vi "Plotter_General.vi"() -> ()   [LabVIEW 2013]
uses:
  Shared/MySQL/Preset Query Enum.ctl
  plotter setup cluster.ctl
  <vilib>/Analysis/NI_AALBase.lvlib
  <vilib>/Analysis/1siggen.llb/Ramp Pattern by Samples.vi
  <vilib>/Utility/tcp.llb/UDP Multicast Read-Only Open.vi
  General-Controler/panel position.ctl
panel:
  in  "STOP button":bool
  in  "shot# 3":i32
  out "error out 3":errorcluster
  out "TCP Ports":refnum<k5>[](array[refnum])
  in  "Device name":string
  in  "shot #":i32
  in  "data string":string
  in  "data string 2":string
  in  "shot # 2":i32
  in  "Device name 2":string
  out "subscribe command":string
  out "size(s)":i32
  out "appended array":string[](array[string])
  out "y2":dbl[](array[numeric])
  out "y1":dbl[](array[numeric])
  out "error out 4":errorcluster
  out "x":dbl[](array[numeric])
  out "portrsvvv":string[](array[string])
  out "ipjjj":string[](array[string])
  out "IPs":string[](array[string])
  out "udp ports to listen to":string[](array[string])
  in  "TCP Open timeout ms":i32=1000
  out "TCP scan error out":errorcluster
  out "ScanData to receive":string[][](array[string])
  out "error out":errorcluster
  in  "Cluster":T1
  out "appargs":string[](array[string])
  out "plotter details":string[][](array[string])
  out "expt":string
  out "Mcast Data":string
  out "TDMS file path":path
  in  "Tab Control 2":T2(tab)
  out "parameters to get":string[][](array[string])
  out "devices to get data from":string[](array[string])
  out "Axis Name List":string[](array[string])
  out "All Devices Core Info":string[][](array[string])
  out "UDP Mcast Error":errorcluster
  in  "Tab Control":T3(tab)=enum."Binned Plot"
  out "xy graph":cluster{dbl[], dbl[]}[](graph)
  out "LHS sigma":dbl format="%_4p"
  out "LHS mean":dbl format="%_4p"
  out "RHS mean":dbl format="%_4p"
  out "RHS sigma":dbl format="%_4p"
  out "Screen\nPosition":cluster{"Left":i16, "Top":i16}
  out "plotter#":string
  out "Scan number":string
  out "xy graph bin":cluster{dbl[], dbl[]}[](graph)=[{[5.5, 15.5, 25.5, 35.5, 45.5, 55.5, 0.0], [0.1, 0.1, 0.15, 0.15, 0.2, 0.2, 0.0]}, {[5.5, 5.5, nan, 15.5, 15.5, nan, 25.5, 25.5, nan, 35.5, 35.5, nan, 45.5, 45.5, nan, 55.5, 55.5, nan, 0.0, 0.0, nan], [0.1, 0.1, nan, 0.1, 0.1, nan, 0.15, 0.15, nan, 0.15, 0.15, nan, 0.2, 0.2, nan, 0.2, 0.2, nan, 0.0, 0.0, nan]}, {[5.5, 15.5, 25.5, 35.5, 45.5, 55.5, 0.0], [5.5, 15.5, 25.5, 35.5, 45.5, 55.5, 0.0]}, {[5.5, 5.5, nan, 15.5, 15.5, nan, 25.5, 25.5, nan, 35.5, 35.5, nan, 45.5, 45.5, nan, 55.5, 55.5, nan, 0.0, 0.0, nan], [3.0, 8.0, nan, 13.0, 18.0, nan, 23.0, 28.0, nan, 33.0, 38.0, nan, 43.0, 48.0, nan, 53.0, 58.0, nan, 0.0, 0.0, nan]}]
  in  "replot":bool
  out "Experiment":u16(ring) items=["Bella", "DataLogging", "HeaterTest", "Lanex Bella", "Plasma2", "Test"]
  out "Current State":string
  out "Mcast Path Data":string
  in  "FilePath":bool
  in  "file path":path
  in  "X Axis":u16(ring)=1 items=["DateTime DateTime shot #", "DateTime Timestamp", "Rep Rate Rep Rate shot #", "Rep Rate Hz"]
  in  "Y Axis":u16(ring) items=["DateTime DateTime shot #", "DateTime Timestamp", "Rep Rate Rep Rate shot #", "Rep Rate Hz"]
  in  "Y Axis 2":u16(ring) items=["DateTime DateTime shot #", "DateTime Timestamp", "Rep Rate Rep Rate shot #", "Rep Rate Hz"]
  out "device data Spreadsheet format":string[][](array[string])
  in  "Left":i16=25
  in  "Top":i16=75
  in  "expt_Plotteridfor vi mode":string="38"
  in  "timeout ms":i32=1000
  out "Actual expt_plotter.id":string
  out "x axis name":string
  out "ScanStart ExptName":string
  out "Y Axis Default name":string
  out "MC_IP":string
  out "Path used":path
  out "error out 2":errorcluster
  out "ScanStatus":string
  in  "data out 1":string
  in  "data out 3":string
  in  "data out 2":string
  out "shotoverride":bool
  in  "shot#":i32
  in  "shot# 2":i32
  out "error out 5":errorcluster
  # "Plotter"
  # "17 Fake cam 1 to 5"
  # "15"
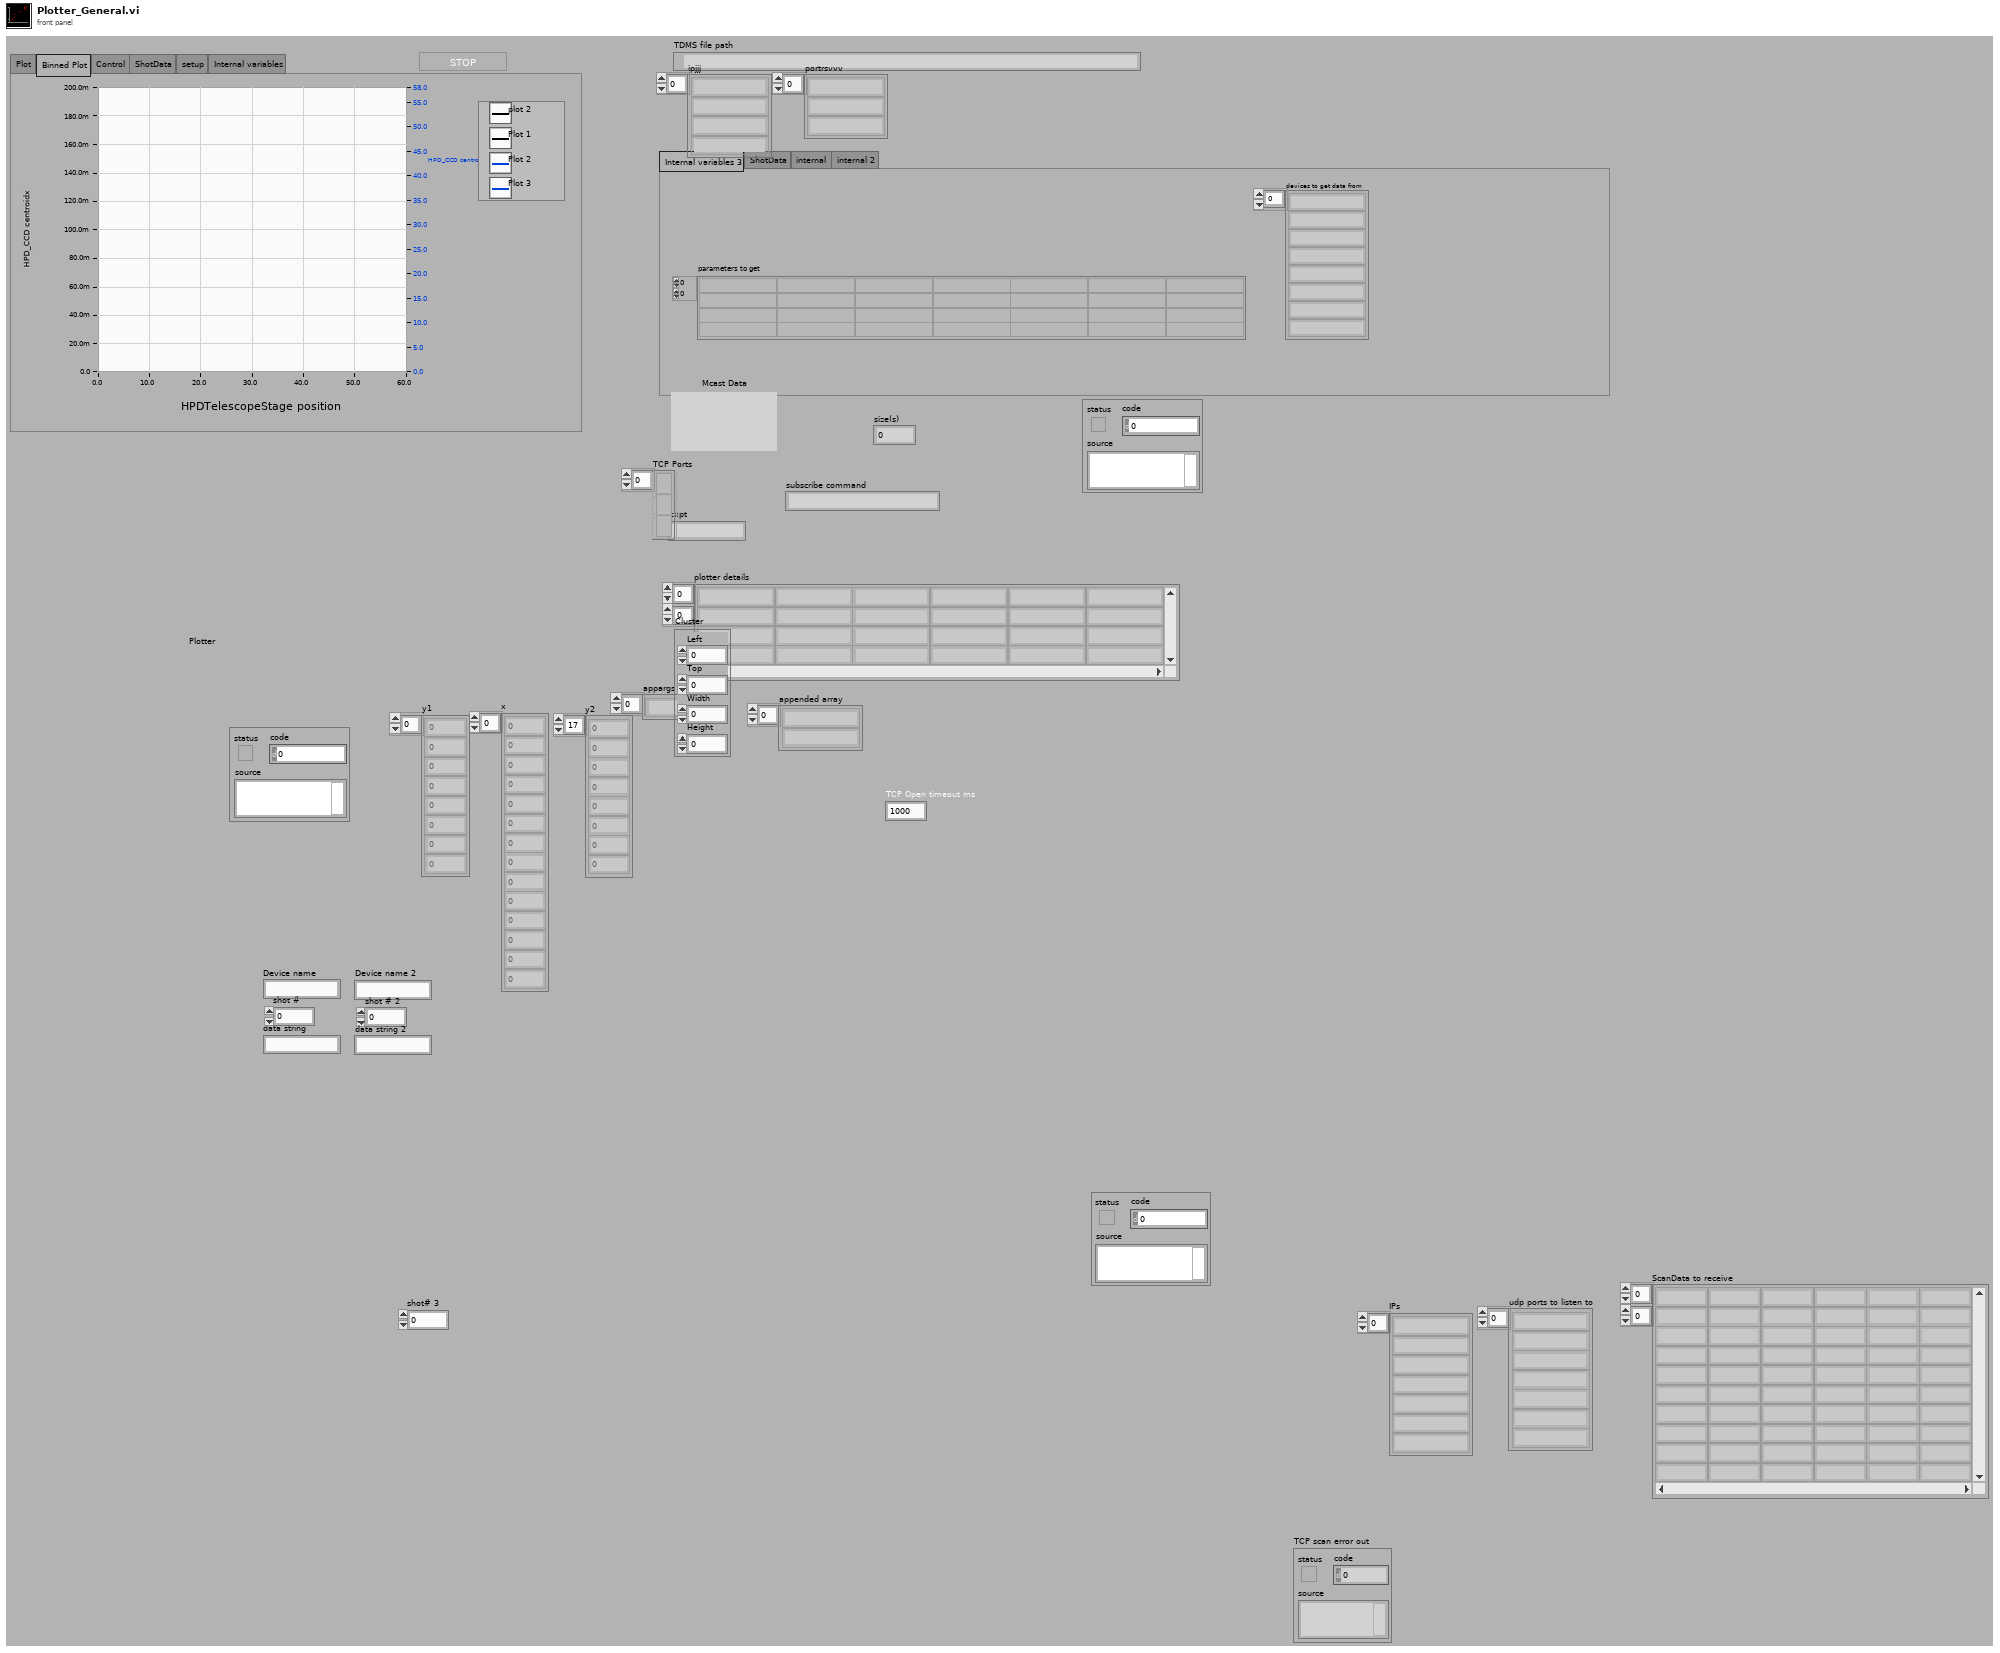
[diagram p1: front panel]
types:
  T1 = typedef "panel position.ctl" = cluster{"Left":i16, "Top":i16, "Width":u32, "Height":u32}
  T2 = enum32{"Internal variables 3", "ShotData", "internal", "internal 2"}
  T3 = enum32{"Plot", "Binned Plot", "Control", "ShotData", "setup", "Internal variables"}
  T4 = typedef "Plotter FGV cluster control.ctl" = cluster{"Multicast Address":string, "Plotter Busy":bool, "Plotter Exit":bool, "Mcast Port":u16}
  T5 = enum32{"invalid app kind", "Development System", "Run Time System", "Student Edition", "Embedded LabVIEW", "Evaluation", "Custom"}
  T6 = enum32{"Invalid", "Standard", "Closed", "Hidden", "Minimized", "Maximized"}
  T7 = typedef "Preset Query Enum.ctl" = enum16{"Get Locations", "Get all IPs and MACs", "Get classes", "Get expt variables to set at scanstart for particular device", "Get expt devices and variables with start values", "Get expt devices and variables (with data to get)", "Get expt devices with data to get", "Get Expt devices and GUIs", "Get all devices basic properties", "Get Virtual Devices Core Info", "Get Expt names", "Get experiment basic properties", "Get experiment alarm variables", "Get MC Ports", "Get device network comm port", "Get devicetype lvclass path", "Get basic device properties", "Get Init Order", "Get all setable variables of a device", "Get device variable aliases", "Get force values of all settable variables", "Get all variables of a devicetype", "Get all variables of a device", "Get plotter details", "Get Saved Scans", "Get Scan Info", "GetGeneralGUIs", "Get expt for plotter", "Get plotter IDs from expt", "Get all devices", "Get all Virtual Devices", "Get all aliases", "Get variable and device info for Virtual Device", "GetItemLocatorIP", "Get IPs for GUIs", "Get DeviceType from Device", "GetLocalPortRange", "GetDevicePresetVariables", "Get Device Configuration", "GetAllPresetNames", "GetAllConfigurationNames", "GetPresetDeviceNames"}
  T8 = typedef "plotter setup cluster.ctl" = cluster{"screenx":i16, "screeny":i16, "variable1":string, "variable2":string, "name":string}
  T9 = cluster{"Ring Refnum x":refnum<vi>, "Ring Refnum y":refnum<vi>, "Ring Refnum y 2":refnum<vi>, "XY Graph Refnum":refnum<vi>}
  T10 = cluster{"Core":cluster{"Current VI Reference":refnum<vi>, "Close Panel on Exit?":bool}, "All Devices Core Info":string[][], "Expt Config Files":string[], "Experiment name":string, "ScanData to receive":string[][], "Device Names for scan data":string[], "expt config file array":string[][], "Data titles from config array":string[], "TDMS file path":path, "Plotter setup cluster":T8, "plotter#":string, "bin complete":bool}
  T11 = typedef "LVRectTypeDef.ctl" = cluster{"Left":i16, "Top":i16, "Right":i16, "Bottom":i16}
  T12 = cluster{"TCP Ports":refnum<vi>, "y1":refnum<vi>, "shot#":refnum<vi>, "data out 1":refnum<vi>}
  T13 = cluster{"TCP Ports":refnum<vi>, "y2":refnum<vi>, "shot# 2":refnum<vi>, "data out 2":refnum<vi>}
  T14 = cluster{"TCP Ports":refnum<vi>, "x":refnum<vi>, "shot# 3":refnum<vi>, "data out 3":refnum<vi>}
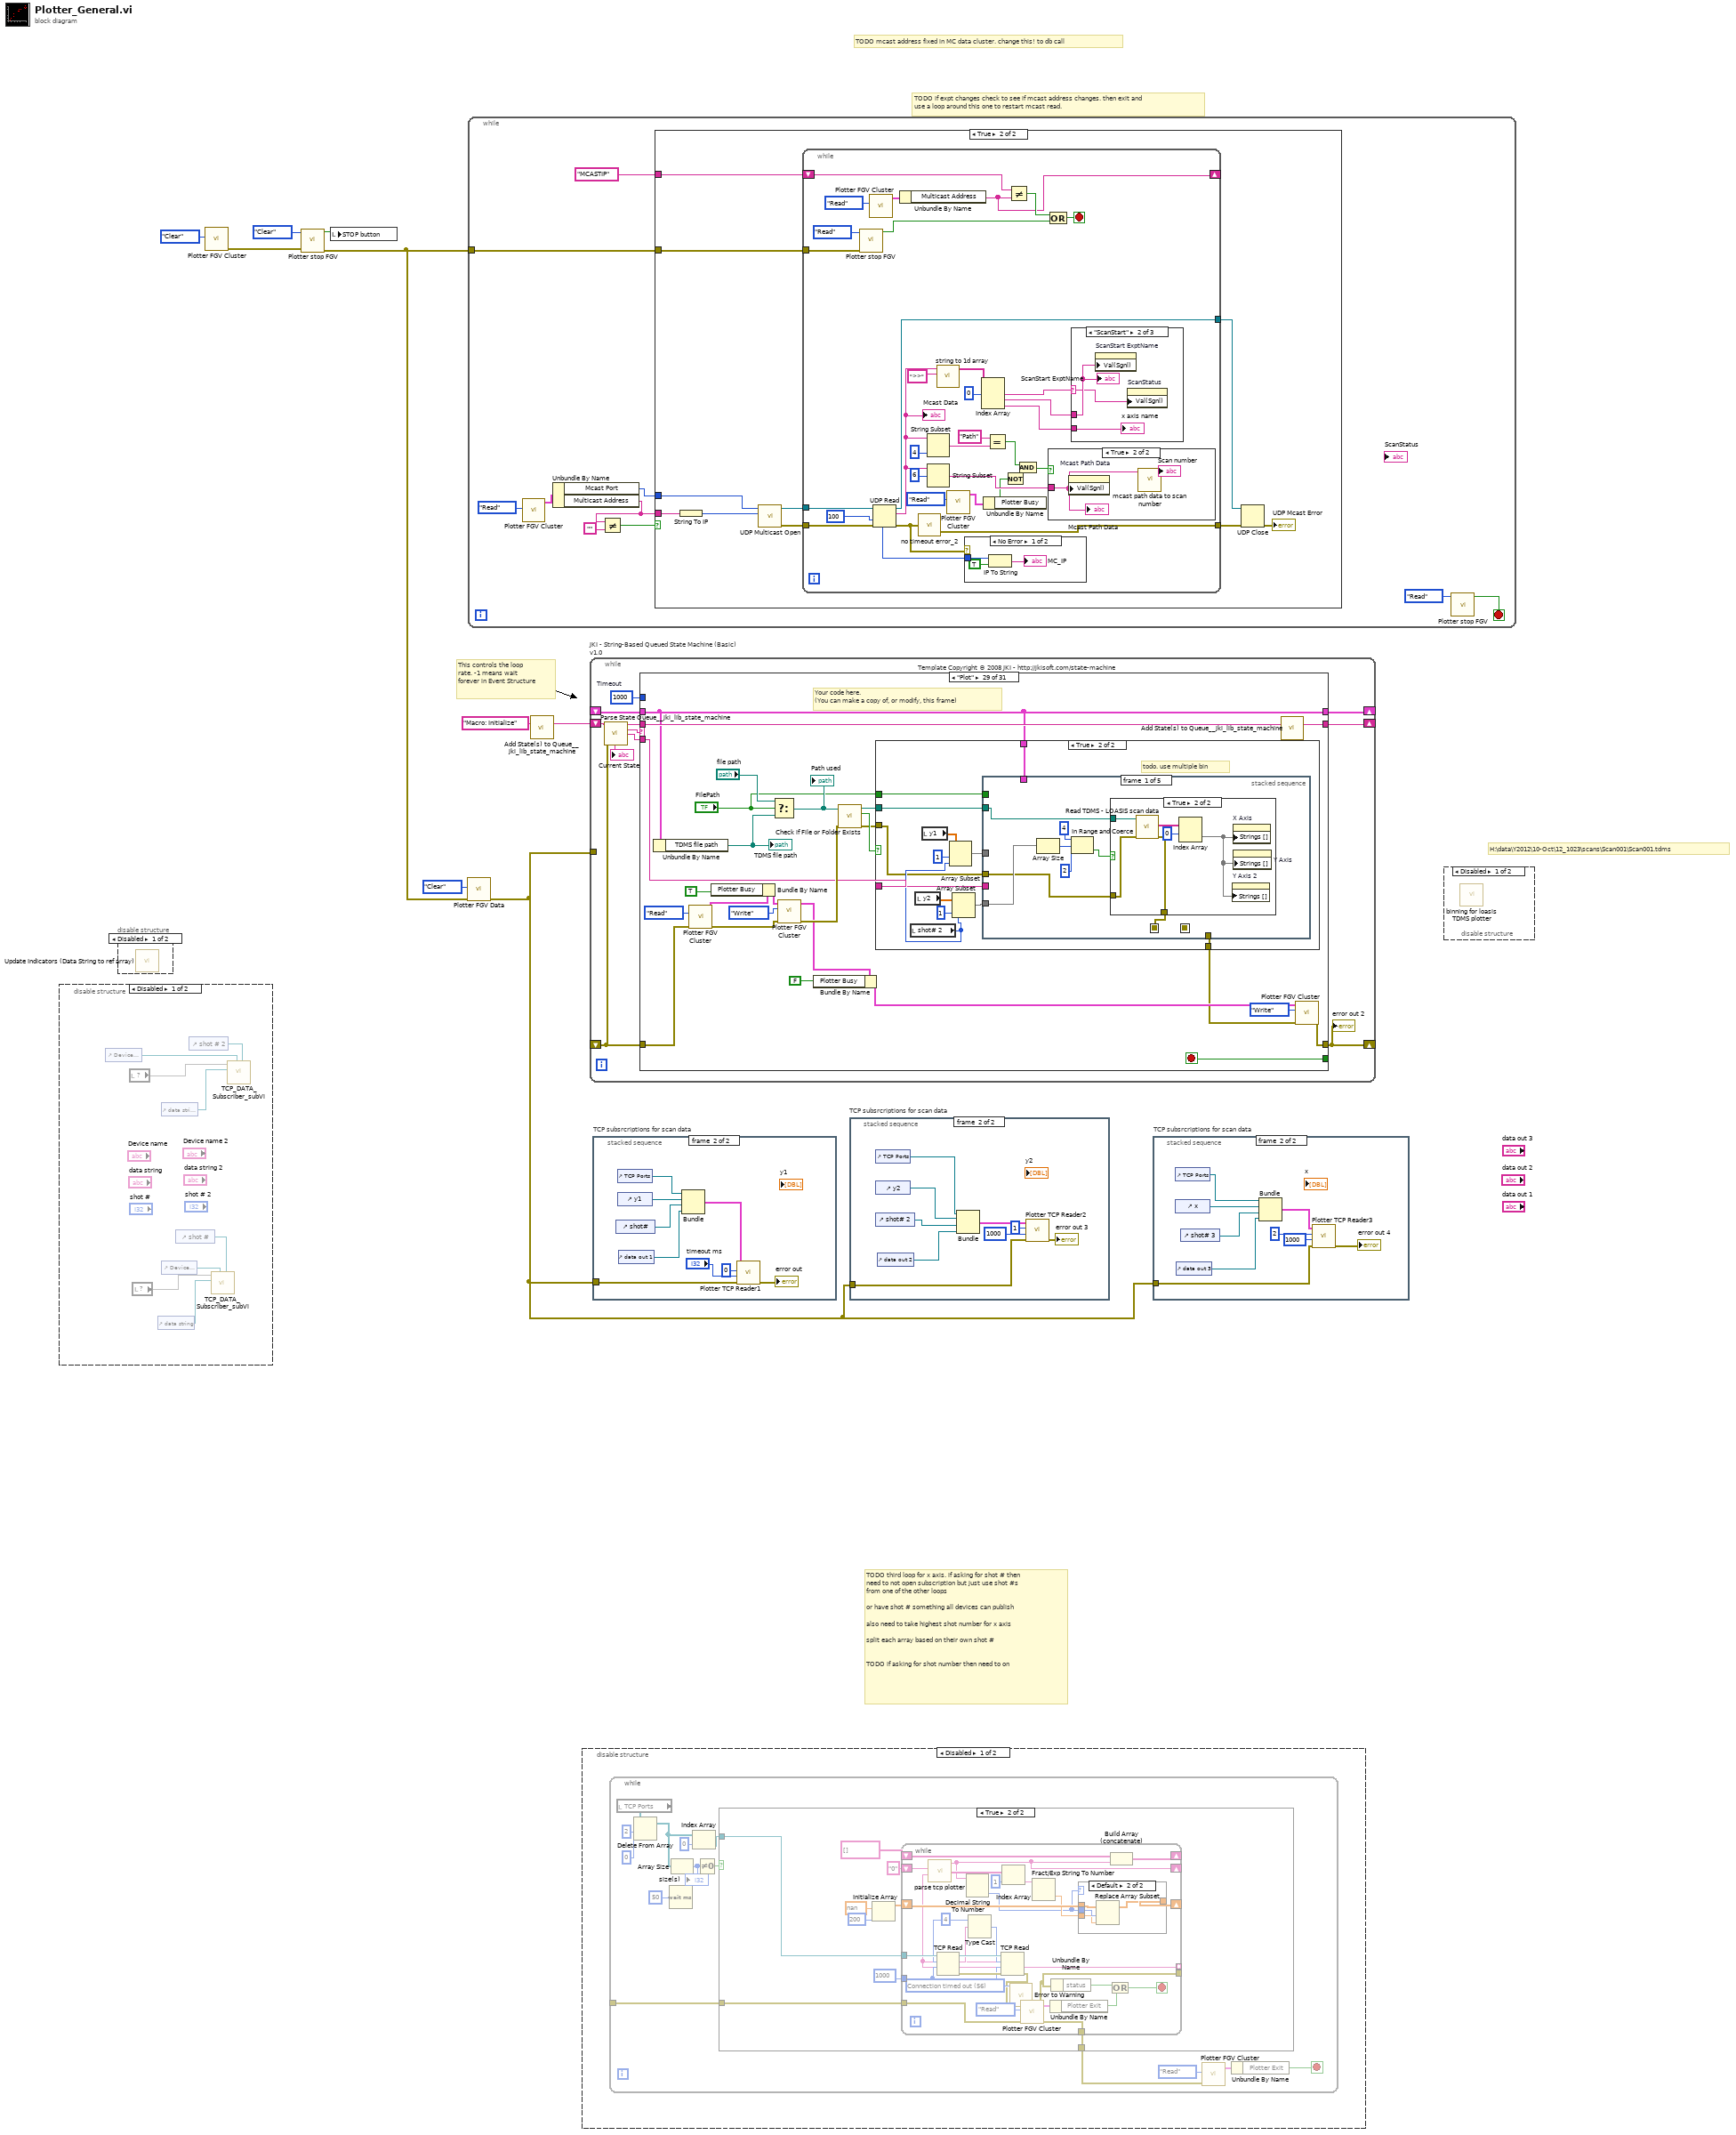
[diagram p0: block diagram]
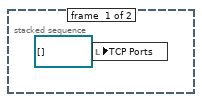
[diagram p6: hidden frame]
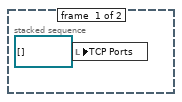
[diagram p7: hidden frame]
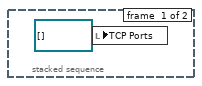
[diagram p9: hidden frame]
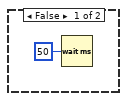
[diagram p11: hidden frame]
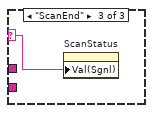
[diagram p15: hidden frame]
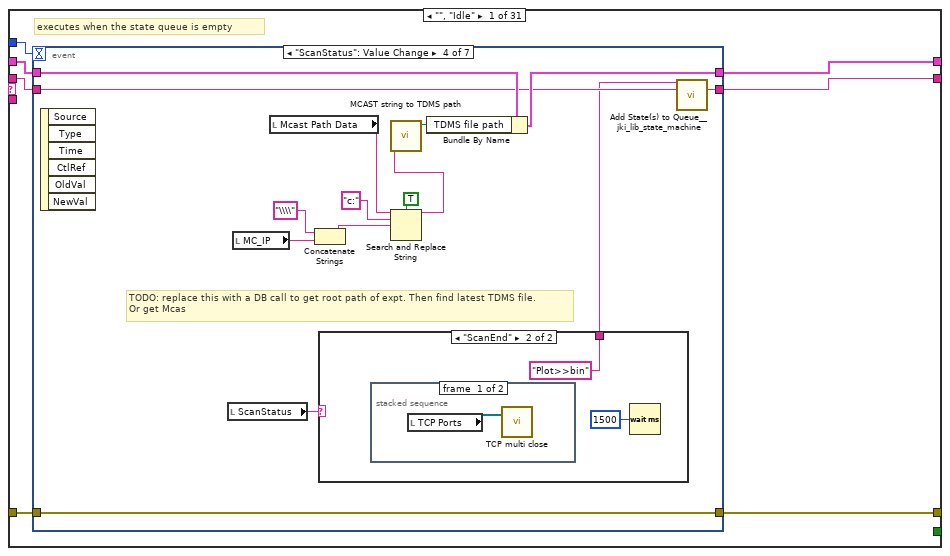
[diagram p16: hidden frame]
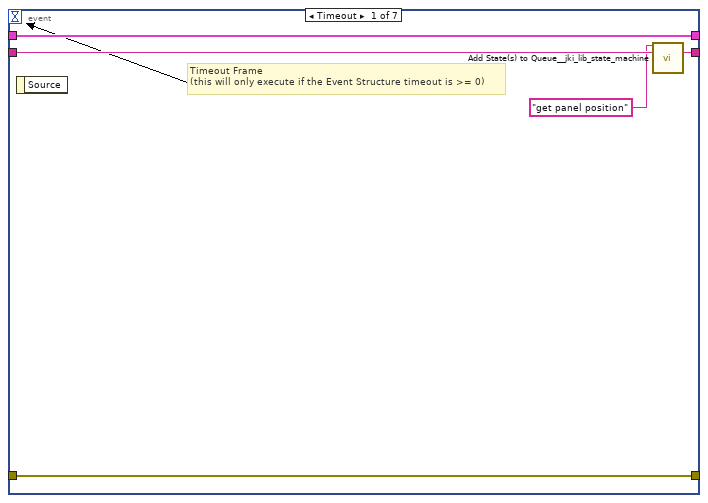
[diagram p17: hidden frame]
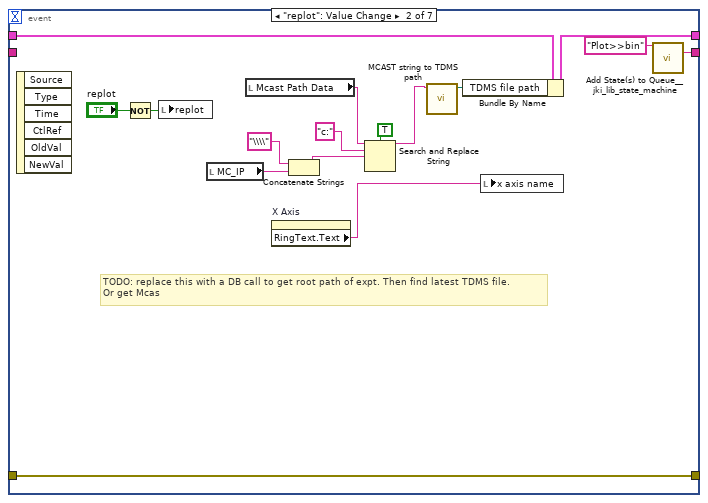
[diagram p18: hidden frame]
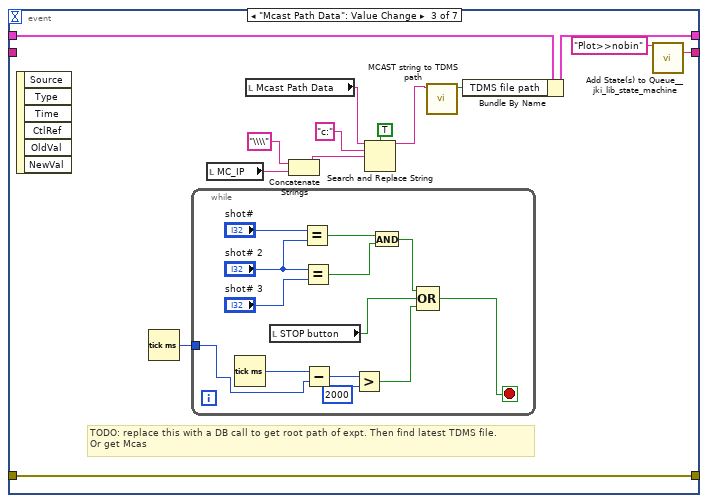
[diagram p19: hidden frame]
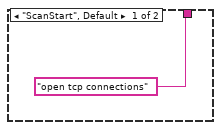
[diagram p20: hidden frame]
diagram:
  # "H:\\data\\Y2012\\10-Oct\\12_1023\\scans\\Scan001\\Scan001.tdms"
  # "TODO third loop for x axis. if asking for shot # then \nneed to not open subscription but just use shot #s\nfrom one of the other loops\n\nor have shot # something all devices can publish\n\nalso need to take highest shot number for x axis\n\nsplit each array based on their own shot #\n\n\nTODO if asking for shot number then need to on"
  # "TODO mcast address fixed in MC data cluster. change this! to db call"
  # "TODO if expt changes check to see if mcast address changes. then exit and\nuse a loop around this one to restart mcast read."
  # "This controls the loop rate. -1 means wait forever in Event Structure"
  n1 = disable-structure shown="Disabled" {
    frame Disabled {
      n2 = control-ref of="Device name 2"() -> (w12:refnum<vi>)
      n3 = local read item#-1() -> (w10)
      n4 = local read item#-1() -> (w15)
      n5 = control-ref of="data string"() -> (w14:refnum<vi>)
      n6 = control-ref of="Device name"() -> (w17:refnum<vi>)
      n7 = control-ref of="data string 2"() -> (w11:refnum<vi>)
      n8 = control-ref of="shot #"() -> (w16:refnum<vi>)
      n9 = control-ref of="shot # 2"() -> (w13:refnum<vi>)
      n10 = call "TCP_DATA_Subscriber_subVi.vi"("shot number"=w16, "whatamI"=w17, 10:w14, "connection ID"=w15) -> ()  [unwired: 7 in, 1 out]
      n11 = call "TCP_DATA_Subscriber_subVi.vi"("shot number"=w13, "whatamI"=w12, 10:w11, "connection ID"=w10) -> ()  [unwired: 7 in, 1 out]
    }
    frame Enabled {
    }
  }
  n12 = disable-structure shown="Disabled" {
    frame Disabled {
      n13 = call "Update Indicators (Data String to ref array).vi"() -> ()  [unwired: 5 in, 1 out]
    }
    frame Enabled {
    }
  }
  n14 = call "Plotter FGV Cluster.vi"("Function"=enum16{"Read", "Write", "Clear"}."Clear") -> ("error out"=w5:errorcluster)  [unwired: 9 in, 1 out]
  n15 = call "Plotter stop FGV.vi"("error in"=w5, "Function"=enum16{"Read", "Write", "Clear"}."Clear") -> ("error out"=w2:errorcluster, "Stop out"=w4:bool)  [unwired: 8 in]
  n16 = local write "STOP button"(w4) -> ()
  n17 = call "Plotter FGV Data.vi"("error in"=w2, "Function"=enum16{"Read", "Write", "Clear"}."Clear") -> ("error out"=w1:errorcluster)  [unwired: 8 in, 1 out]
  n18 = while {
    tunnel: w2 -> [w21]
    stop <- w25 stop-if-true
    n19 = call "Plotter FGV Cluster.vi"("Function"=enum16{"Read", "Write", "Clear"}."Read") -> ("Cluster out"=w22:T4)  [unwired: 9 in, 1 out]
    n20 = Unbundle By Name(w22) -> ("Mcast Port"=w18:u16, "Multicast Address"=w20:string)
    n21 = Not Equal?(x=w20, y="") -> (x != y?=w24:bool)
    n22 = case shown="True" w24 {
      tunnel: "MCASTIP" ("Multicast Address") -> [_ w32]
      tunnel: w20 -> [_ w31]
      tunnel: w21 -> [_ w30]
      tunnel: w18 -> [_ w29]
      frame False {
        n23 = Wait (ms)(milliseconds to wait=u32 50) -> ()  [unwired: 1 out]
      }
      frame True {
        n24 = String To IP(1:w31) -> (0:w38:u32)
        n25 = call-poly <vilib>:"UDP Multicast Open.vi"("multicast addr"=w38, "port"=w29) -> ("error out"=w33:errorcluster, "connection ID"=w37:refnum<k16>)  [unwired: 7 in, 1 out]
        n26 = while {
          tunnel: w37 -> [w71]
          tunnel: [w70] -> w36
          tunnel: [w69] -> w35
          tunnel: w33 -> [w65]
          tunnel: w30 -> [w63]
          shift-right: [w39] -> _
          shift-left: w32 -> [w51]
          stop <- w52 stop-if-true
          n27 = call "Plotter stop FGV.vi"("error in"=w63, "Function"=enum16{"Read", "Write", "Clear"}."Read") -> ("Stop out"=w53:bool)  [unwired: 8 in, 1 out]
          n28 = call "Plotter FGV Cluster.vi"("Function"=enum16{"Read", "Write", "Clear"}."Read") -> ("Cluster out"=w50:T4)  [unwired: 9 in, 1 out]
          n29 = UDP Read(connection ID=w71, timeout ms (25000)=100, 8:w65) -> (data out=w54:string, error out=w41:errorcluster, 3:w70:refnum<k16>, 6:w42:u32)  [unwired: 2 out]
          "Mcast Data" <- w54
          n30 = Unbundle By Name(w50) -> ("Multicast Address"=w39:string)
          n31 = call "no timeout error_2.vi"("error in (no error)"=w41) -> ("error out"=w69:errorcluster)  [unwired: 1 out]
          n32 = String Subset(string=w54, length (rest)=4 ("length (rest)")) -> (substring=w60:string)  [unwired: 1 in]
          n33 = String Subset(string=w54, offset (0)=6) -> (substring=w58:string)  [unwired: 1 in]
          n34 = call "string to 1d array.vi"("delimiter (Tab)"=">>", "string"=w54) -> ("Array of Strings"=w67:string[])  [unwired: 9 in]
          n35 = call "Plotter FGV Cluster.vi"("Function"=enum16{"Read", "Write", "Clear"}."Read") -> ("Cluster out"=w45:T4)  [unwired: 9 in, 1 out]
          n36 = case shown="No Error" w41 {
            tunnel: w42 -> [w75 _]
            frame No Error {
              n37 = IP To String(1:TRUE ("dot notation? (F)"), 2:w75) -> (0:→"MC_IP":string)
            }
            frame Error {
            }
          }
          n38 = Index Array(array=w67, index #1=0 ("index")) -> (element #1=w48:string, element #2=w55:string, element #3=w56:string)  [unwired: 2 in]
          n39 = Unbundle By Name(w45) -> ("Plotter Busy"=w44:bool)
          n40 = Equal?(x="Path" ("y"), y=w60) -> (x = y?=w57:bool)
          n41 = Not(x=w44) -> (.not. x?=w43:bool)
          n42 = Not Equal?(x=w51, y=w39) -> (x != y?=w40:bool)
          n43 = And(x=w57, y=w43) -> (x .and. y?=w47:bool)
          n44 = case shown="True" w47 {
            tunnel: w58 -> [_ w77]
            frame False {
            }
            frame True {
              n45 = property on="Mcast Path Data" class="Str"("Val(Sgnl)"=w77) -> ()  [unwired: 2 in, 2 out]
              n46 = call "mcast path data to scan number.vi"("mcast path data"=w77) -> ("Scan number"=→"Scan number":string)  [unwired: 10 in]
              "Mcast Path Data" <- w77
            }
          }
          n47 = Compound Arithmetic op=OR(w40, w53) -> (w52:bool)
          n48 = case shown="\"ScanStart\"" w48 {
            selector: w48 -> [_ w78 w81]
            tunnel: w56 -> [_ w80 _]
            tunnel: w55 -> [_ w79 _]
            frame Default {
            }
            frame "ScanStart" {
              n49 = property on="ScanStart ExptName" class="Str"("Val(Sgnl)"=w79) -> ()  [unwired: 2 in, 2 out]
              n50 = property on="ScanStatus" class="Str"("Val(Sgnl)"=w78) -> ()  [unwired: 2 in, 2 out]
              "x axis name" <- w80
              "ScanStart ExptName" <- w79
            }
            frame "ScanEnd" {
              n51 = property on="ScanStatus" class="Str"("Val(Sgnl)"=w81) -> ()  [unwired: 2 in, 2 out]
            }
          }
        }
        n52 = UDP Close(connection ID=w36, 8:w35) -> (error out=→"UDP Mcast Error":errorcluster)  [unwired: 1 out]
      }
    }
    n53 = call "Plotter stop FGV.vi"("Function"=enum16{"Read", "Write", "Clear"}."Read") -> ("Stop out"=w25:bool)  [unwired: 9 in, 1 out]
  }
  n54 = call <vilib>:"Add State(s) to Queue__jki_lib_state_machine.vi"("State(s) in (\"\")"="Macro: Initialize") -> ("States Out"=w9:string)  [unwired: 14 in]
  n55 = disable-structure shown="Disabled" {
    frame Disabled {
      n56 = while {
        tunnel: _ -> [w88]
        stop <- w89 stop-if-true
        n57 = local read "TCP Ports"() -> (w92:refnum<k5>[])
        n58 = Delete From Array(array=w92, length=2, index=0) -> (array with subset deleted=w84:refnum<k5>[])  [unwired: 1 out]
        n59 = Wait (ms)(milliseconds to wait=u32 50) -> ()  [unwired: 1 out]
        n60 = Array Size(array=w84) -> (size(s)=w95:i32)
        "size(s)" <- w95
        n61 = Index Array(array=w84, index=0) -> (element=w87:refnum<k5>)
        n62 = Not Equal To 0?(x=w95) -> (x != 0?=w94:bool)
        n63 = case shown="True" w94 {
          tunnel: w87 -> [_ w103]
          tunnel: w88 -> [_ w102]
          tunnel: [_ w101] -> w82
          frame False {
          }
          frame True {
            n64 = Initialize Array(nan ("element"), 200 ("dimension size")) -> (w96:dbl[])
            n65 = while {
              tunnel: [w114] -> _
              tunnel: w103 -> [w132]
              tunnel: 1000 ("timeout ms 3") -> [w130]
              tunnel: [w105] -> _ mode=indexing
              shift-right: [w113] -> _
              shift-left: "0" ("shot #") -> [w124]
              tunnel: w102 -> [w120]
              tunnel: [w119] -> w101
              shift-right: [w111] -> _
              shift-left: string[] [] -> [w112]
              shift-right: [w107] -> _
              shift-left: w96 -> [w109]
              stop <- w126 stop-if-true
              w116 = 56 items=["No Error", "Argument Error", "Memory Full", "Out of Zone", "End of File", "File Already Open", "Generic File IO Error", "File Not Found", "File Permission Error", "Disk Full", "Duplicate Path", "Too Many Files Open", "Not Enabled", "Resource File Not Found", "Cannot Add Resource", "Resource Not Found", "Image Not Found", "Image Memory Error", "Pen Does Not Exist", "Config Bad Type", "Config Token Not Found", "Config Parse Error", "Config Memory Error", "Bad External Code Format", "Bad External Code Offset", "External Code Not Present", "Null Window", "Destroy Window Mixup", "Null Menu", "Print Aborted", "Bad Print Record", "Print Driver Error", "Windows Error During Print", "Memory Error During Print", "Print Dialog Error", "Generic Print Error", "Invalid Device Refnum", "Device Not Found", "Device Parameter Error", "Device Unit Error", "Can't Open Device", "Device Call Aborted", "Generic Error", "Cancelled By User", "Object ID Too Low", "Object ID Too High", "Object Not In Heap", "Unknown Heap", "Bad DefProc ID", "DefProc Not In Table", "Message Out Of Range", "Null Method", "Unknown Message", "Manager Call Not Supported", "Bad address", "Connection In progress", "Connection timed out", "Connection is already in progress", "Network attribute not supported", "Network error", "Address in use", "System out of memory", "Connection aborted", "Connection refused", "Connection is not connected", "Connection is already connected", "Connection closed", "Initialize error (interapplication manager)", "Bad occurrence", "Wait on unbound occurrence handler", "Occurrence queue overflow", "Bad path", "Semaphore not signaled", "Unrecognized type (interapplication manager)"] ("1st Error to Convert")
              w129 = 4 ("bytes to read")
              n66 = TCP Read(connection ID=w132, bytes to read=w129, 9:w130) -> (connection ID out=w133:refnum<k5>, data out=w128:string, error out=w131:errorcluster)  [unwired: 2 in]
              n67 = Type Cast(type=w129, x=w128) -> (*(type *) &x=w127:i32)
              n68 = TCP Read(connection ID=w133, bytes to read=w127, error in (no error)=w131, 9:w130) -> (data out=w105:string, error out=w115:errorcluster)  [unwired: 1 in, 1 out]
              n69 = call "parse tcp plotter.vi"("data in"=w105, "shot #"=w124) -> ("variable values"=w118:string[], "shot # out"=w113:string)  [unwired: 8 in]
              n70 = Decimal String To Number(string=w113) -> (number=w106:i32)  [unwired: 2 in, 1 out]
              n71 = Index Array(array=w118, index=1) -> (element=w117:string)
              n72 = call <vilib>:"Error to Warning.vi"("1st Error to Convert"=w116, "error in"=w115) -> ("warning out"=w114:errorcluster)  [unwired: 13 in]
              n73 = call "Plotter FGV Cluster.vi"("error in"=w120, "Function"=enum16{"Read", "Write", "Clear"}."Read") -> ("error out"=w119:errorcluster, "Cluster out"=w122:T4)  [unwired: 8 in]
              n74 = Fract/Exp String To Number(string=w117) -> (number=w108:dbl)  [unwired: 3 in, 1 out]
              n75 = Unbundle By Name(w122) -> ("Plotter Exit"=w121:bool)
              n76 = Unbundle By Name(w114) -> ("status"=w125:bool)
              n77 = case shown="Default" w106 {
                tunnel: w109 -> [w134 w138]
                tunnel: w106 -> [_ w137]
                tunnel: w108 -> [_ w136]
                tunnel: [w134 w135] -> w107
                frame 0 {
                }
                frame Default {
                  n78 = Replace Array Subset(array=w138, new element=w136, index=w137) -> (w135:dbl[])
                }
              }
              n79 = Or(x=w125, y=w121) -> (x .or. y?=w126:bool)
              n80 = Build Array (concatenate)(w112, w113) -> (w111:string[])
            }
          }
        }
        n81 = call "Plotter FGV Cluster.vi"("error in"=w82, "Function"=enum16{"Read", "Write", "Clear"}."Read") -> ("Cluster out"=w91:T4)  [unwired: 8 in, 1 out]
        n82 = Unbundle By Name(w91) -> ("Plotter Exit"=w89:bool)
      }
    }
    frame Enabled {
    }
  }
  n83 = while "JKI - String-Based Queued State Machine (Basic) v1.0" {
    shift-right: [w143] -> _
    shift-left: _ -> [w142]
    shift-right: [w139] -> _
    shift-left: _ -> [w140]
    shift-right: [w145] -> _
    shift-left: w9 -> [w146]
    tunnel: w1 -> [_]
    stop <- w144 stop-if-true
    w141 = 1000  # Timeout
    # "Template Copyright © 2008 JKI - http://jkisoft.com/state-machine"
    n84 = call <vilib>:"Parse State Queue__jki_lib_state_machine.vi"("State Queue"=w146, "Error In (no error)"=w140) -> ("Remaining States"=w148:string, "Current State"=w149:string, "Arguments"=w147:string)  [unwired: 11 in]
    "Current State" <- w149
    n85 = case shown="\"Plot\"" w149 {
      selector: w149 -> [_ _ _ w264 _ _ _ _ _ _ _ _ _ _ _ _ _ _ _ _ _ _ _ _ _ _ _ _ _ _ _]
      tunnel: w148 -> [w156 w259 w263 w268 w286 w293 w298 w302 w306 w312 w316 w320 w326 w337 w363 w368 w378 w382 w388 w397 w417 w446 w475 w488 w504 w519 w592 w600 w625 w737 w747]
      tunnel: w147 -> [_ _ _ _ _ _ _ _ _ _ _ _ w321 w331 _ _ _ _ _ _ _ _ _ _ _ _ _ _ w603 _ _]
      tunnel: w142 -> [w154 w256 w260 w266 w277 w290 w296 w299 _ w307 w313 w318 w324 w333 w360 w364 w376 w379 w385 w394 w415 w432 w473 w481 w501 w517 w586 w597 w623 w734 w745]
      tunnel: [w153 w257 w261 w270 w283 errorcluster {"status"=FALSE, "code"=0, "source"=""} ("error out") w295 w300 w304 w308 w314 w317 w322 w334 w361 w366 w369 w380 w386 w389 w403 w428 w464 w486 w502 w515 w577 w593 w604 w735 w742] -> w139
      tunnel: w140 -> [w152 w257 w261 w269 w283 w287 w295 w300 w304 w309 w314 w317 w323 w335 w361 w366 w369 w380 w386 w390 w404 w429 w454 w486 w502 w516 w578 w594 w605 w735 w743]
      tunnel: [w155 w258 w262 w267 w285 w292 w297 w301 w305 w311 w315 w319 w325 w336 w362 w367 w377 w381 w387 w396 w416 w445 w474 w487 w503 w518 w591 w599 w624 w736 w746] -> w145
      tunnel: [_ _ _ _ _ _ TRUE _ _ _ _ _ _ _ _ _ _ _ _ _ _ _ _ _ _ _ _ _ _ _ _] -> w144
      tunnel: [w151 w256 w260 w266 w284 w290 w296 w299 w303 w307 w313 w318 w324 w333 w360 w364 w376 w379 w385 w393 w414 w431 w472 w480 w501 w517 w586 w598 w623 w734 w745] -> w143
      tunnel: w141 -> [w150 _ _ _ _ _ _ _ _ _ _ _ _ _ _ _ _ _ _ _ _ _ _ _ _ _ _ _ _ _ _]
      frame "", "Idle" {
        # "executes when the state queue is empty"
        n86 = event shown="[3] \"ScanStatus\": Value Change" {
          selector: _ -> [_ _ _ _ _ _ _]
          dyn-events: _ -> [_ _ _ _ _ _ _]
          timeout: w150 -> [_ _ _ _ _ _ _]
          tunnel: w156 -> [w161 _ _ w214 w235 w249 w255]
          tunnel: [w160 w177 w191 w219 w234 w248 w254] -> w155
          tunnel: w154 -> [w158 w174 w188 w217 w226 w246 w252]
          tunnel: [w159 w176 w190 w218 w233 w247 w253] -> w153
          tunnel: w152 -> [w159 w176 w190 w218 w233 w247 w253]
          tunnel: [w158 w173 w187 w216 w225 w246 w252] -> w151
          event Timeout {
            # "Timeout Frame\n(this will only execute if the Event Structure timeout is >= 0)"
            n87 = event-data() -> ()  [unwired: 1 in, 1 out]
            n88 = call <vilib>:"Add State(s) to Queue__jki_lib_state_machine.vi"("State(s) in Front (\"\")"="get panel position", "State(s) in (\"\")"=w161) -> ("States Out"=w160:string)  [unwired: 13 in]
          }
          event "replot": Value Change {
            # "TODO: replace this with a DB call to get root path of expt. Then find latest TDMS file.\nOr get Mcas"
            n89 = event-data() -> ()  [unwired: 1 in, 6 out]
            n90 = Not(x="replot") -> (.not. x?=w171:bool)
            n91 = local write "replot"(w171) -> ()
            n92 = local read "MC_IP"() -> (w167:string)
            n93 = local read "Mcast Path Data"() -> (w169:string)
            n94 = property on="X Axis" class="Ring (strict)"() -> ("RingText.Text"=w162:string)  [unwired: 2 in, 2 out]
            n95 = Concatenate Strings("\\\\" ("string"), w167) -> (w164:string)
            n96 = Search and Replace String(case sensitive?=TRUE ("ignore case? (F)"), input string=w169, search string="c:" ("string"), replace string=w164) -> (result string=w163:string)  [unwired: 4 in, 3 out]
            n97 = call "MCAST string to TDMS path.vi"("MCAST path"=w163) -> ("TDMS path"=w170:path)  [unwired: 10 in]
            n98 = Bundle By Name(cluster=w174, "TDMS file path"=w170) -> (w173:T10)
            n99 = local write "x axis name"(w162) -> ()
            n100 = call <vilib>:"Add State(s) to Queue__jki_lib_state_machine.vi"("State(s) in Front (\"\")"="Plot>>bin" ("State(s) in Front (\"\")")) -> ("States Out"=w177:string)  [unwired: 14 in]
          }
          event "Mcast Path Data": Value Change {
            # "TODO: replace this with a DB call to get root path of expt. Then find latest TDMS file.\nOr get Mcas"
            n101 = event-data() -> ()  [unwired: 1 in, 6 out]
            n102 = Tick Count (ms)() -> (millisecond timer value=w178:u32)
            n103 = while {
              tunnel: w178 -> [w196]
              stop <- w192 stop-if-true
              n104 = Tick Count (ms)() -> (millisecond timer value=w197:u32)
              n105 = local read "STOP button"() -> (w198:bool)
              n106 = Equal?(x="shot#", y="shot# 2") -> (x = y?=w201:bool)
              n107 = Equal?(x="shot# 2", y="shot# 3") -> (x = y?=w204:bool)
              n108 = Subtract(x=w197, y=w196) -> (x-y=w195:u32)
              n109 = Greater?(x=w195, y=u32 2000) -> (0:w193:bool)
              n110 = And(x=w201, y=w204) -> (x .and. y?=w199:bool)
              n111 = Compound Arithmetic op=OR(w199, w198, w193) -> (w192:bool)
            }
            n112 = local read "MC_IP"() -> (w183:string)
            n113 = local read "Mcast Path Data"() -> (w185:string)
            n114 = Concatenate Strings("\\\\" ("string"), w183) -> (w180:string)
            n115 = Search and Replace String(case sensitive?=TRUE ("ignore case? (F)"), input string=w185, search string="c:" ("string"), replace string=w180) -> (result string=w179:string)  [unwired: 4 in, 3 out]
            n116 = call "MCAST string to TDMS path.vi"("MCAST path"=w179) -> ("TDMS path"=w186:path)  [unwired: 10 in]
            n117 = Bundle By Name(cluster=w188, "TDMS file path"=w186) -> (w187:T10)
            n118 = call <vilib>:"Add State(s) to Queue__jki_lib_state_machine.vi"("State(s) in Front (\"\")"="Plot>>nobin" ("State(s) in Front (\"\")")) -> ("States Out"=w191:string)  [unwired: 14 in]
          }
          event "ScanStatus": Value Change {
            # "TODO: replace this with a DB call to get root path of expt. Then find latest TDMS file.\nOr get Mcas"
            n119 = event-data() -> ()  [unwired: 1 in, 6 out]
            n120 = local read "ScanStatus"() -> (w206:string)
            n121 = local read "MC_IP"() -> (w212:string)
            n122 = local read "Mcast Path Data"() -> (w208:string)
            n123 = Concatenate Strings("\\\\" ("string"), w212) -> (w209:string)
            n124 = case shown="\"ScanEnd\"" w206 {
              tunnel: ["open tcp connections" ("State(s) in Front (\"\")") "Plot>>bin" ("State(s) in Front (\"\")")] -> w205
              frame "ScanStart", Default {
              }
              frame "ScanEnd" {
                n125 = stacked-sequence {
                  frame #0 {
                    n126 = local read "TCP Ports"() -> (w223:refnum<k5>[])
                    n127 = call "TCP multi close.vi"("TCP Ports"=w223) -> ()  [unwired: 2 in, 1 out]
                  }
                  frame #1 {
                    n128 = local write "TCP Ports"(refnum<k5>[] [] ("TCP Ports")) -> ()
                  }
                }
                n129 = Wait (ms)(milliseconds to wait=u32 1500) -> ()  [unwired: 1 out]
              }
            }
            n130 = Search and Replace String(case sensitive?=TRUE ("ignore case? (F)"), input string=w208, search string="c:" ("string"), replace string=w209) -> (result string=w207:string)  [unwired: 4 in, 3 out]
            n131 = call "MCAST string to TDMS path.vi"("MCAST path"=w207) -> ("TDMS path"=w215:path)  [unwired: 10 in]
            n132 = Bundle By Name(cluster=w217, "TDMS file path"=w215) -> (w216:T10)
            n133 = call <vilib>:"Add State(s) to Queue__jki_lib_state_machine.vi"("State(s) in Front (\"\")"=w205, "State(s) in (\"\")"=w214) -> ("States Out"=w219:string)  [unwired: 13 in]
          }
          event "ScanStart ExptName": Value Change {
            w228 = dbl[] [] ("y1")
            n134 = event-data() -> ()  [unwired: 1 in, 6 out]
            n135 = Bundle By Name(cluster=w226, "bin complete"=FALSE) -> (w225:T10)
            n136 = local read "ScanStart ExptName"() -> (w230:string)
            n137 = property on="Experiment" class="Ring (strict)"() -> ("Strings []"=w231:string[])  [unwired: 2 in, 2 out]
            n138 = Search 1D Array(1D array=w231, element=w230) -> (index of element=w229:i32)  [unwired: 1 in]
            n139 = local write "y2"(w228) -> ()
            n140 = local write "y1"(w228) -> ()
            n141 = local write "x"(w228) -> ()
            n142 = local write "Experiment"(w229) -> ()
            n143 = call <vilib>:"Add State(s) to Queue__jki_lib_state_machine.vi"("State(s) in Front (\"\")"="Main: Macro", "State(s) in (\"\")"=w235) -> ("States Out"=w234:string)  [unwired: 13 in]
          }
          event "STOP button": Value Change {
            # "Exit Button Value Change (pressed) Event\n(this executes Macro: Exit to terminate the VI)"
            n144 = event-data() -> ()  [unwired: 1 in, 1 out]
            n145 = call "Plotter stop FGV.vi"("Stop in"="STOP button", "Function"=enum16{"Read", "Write", "Clear"}."Write") -> ("Stop out"=w243:bool)  [unwired: 8 in, 1 out]
            n146 = Not(x=w243) -> (.not. x?=w242:bool)
            n147 = call "Plotter FGV Cluster.vi"("Function"=enum16{"Read", "Write", "Clear"}."Read") -> ("Cluster out"=w238:T4)  [unwired: 9 in, 1 out]
            n148 = Bundle By Name(cluster=w238, "Plotter Exit"=TRUE) -> (w236:T4)
            n149 = local write "STOP button"(w242) -> ()
            n150 = call "Plotter FGV Cluster.vi"("Function"=enum16{"Read", "Write", "Clear"}."Write", "Cluster in"=w236) -> ()  [unwired: 8 in, 2 out]
            n151 = call <vilib>:"Add State(s) to Queue__jki_lib_state_machine.vi"("State(s) in Front (\"\")"="Macro: Exit", "State(s) in (\"\")"=w249) -> ("States Out"=w248:string)  [unwired: 13 in]
          }
          event Panel Close? {
            # "Discard the event because we'll close the front panel ourselves in Macro: Exit"
            # "Close Panel button (pressed) Event\n(this executes Macro: Exit to terminate the VI)"
            n152 = event-data() -> ()  [unwired: 1 in, 1 out]
            n153 = event-data("Discard?"=TRUE) -> ()  [unwired: 1 in, 1 out]
            n154 = call <vilib>:"Add State(s) to Queue__jki_lib_state_machine.vi"("State(s) in Front (\"\")"="Macro: Exit", "State(s) in (\"\")"=w255) -> ("States Out"=w254:string)  [unwired: 13 in]
          }
        }
      }
      frame "Readme" {
        # "For instructions on how to use the JKI State Machine, examples and video tutorials, visit:\nhttp://jkisoft.com/state-machine/\n\nJKI State Machine™\nhttp://jkisoft.com/state-machine/\nCopyright (C) 2005-2008, JKI <info@jkisoft.com>\nALL RIGHTS RESERVED"
        # "copy this to create labels for wires"
        # "System_Label"
        # "State Syntax:\nStateCategory: State >> Argument\nLine Terminator: Line feed\nExample:\nUI: Help >> About\n\nWhere \"UI\" is the state category\nWhere \"Help\" is the state\nWhere \"About\" is the argument\nOther Examples:\nApp Data: Initialize\nUI: Initialize\nHelp >> About\n\nCommenting:\nTo add a comment use \"//\" or \"#\" and all text to the right will be ignored\nCommenting Example:\nUI: Initialize // This initializes the UI\n# This whole line is a comment\n// Another comment line"
        # "Readme"
        n155 = call <vilib>:"Add State(s) to Queue__jki_lib_state_machine.vi"("State(s) in (\"\")"=w259) -> ("States Out"=w258:string)  [unwired: 14 in]
      }
      frame "---------- Core ----------" {
        # "Do not put any code in this frame.\n(it is a separator no-op)"
        n156 = call <vilib>:"Add State(s) to Queue__jki_lib_state_machine.vi"("State(s) in (\"\")"=w263) -> ("States Out"=w262:string)  [unwired: 14 in]
      }
      frame Default {
        w273 = 42 items=["No error", "Argument error", "Memory is full", "Out of zone", "End of file", "File already open", "Generic file I/O error", "File not found", "File permission error", "Disk is full", "Duplicate path", "Too many files open", "System feature not enabled", "Resource file not found", "Cannot add resource", "Resource not found", "Image not found", "Image memory error", "Pen does not exist", "Config type invalid", "Config token not found", "Config parse error", "Config memory error", "Bad external code format", "Bad external code offset", "External code not present", "Null window", "Destroy window error", "Null menu", "Print aborted", "Bad print record", "Print driver error", "Windows error during printing", "Memory error during printing", "Print dialog error", "Generic print error", "Invalid device refnum", "Device not found", "Device parameter error", "Device unit error", "Cannot open device", "Device call aborted", "Generic error", "Cancelled by user", "Object ID too low", "Object ID too high", "Object not in heap", "Unknown heap", "Unknown object (invalid DefProc)", "Unknown object (DefProc not in table)", "Message out of range", "Invalid (null) method", "Unknown message", "Manager call not supported", "Bad address", "Network operation in progress", "Network operation timed out", "Connection is busy", "Network attribute not supported", "Network error", "Address in use", "System out of memory", "Connection aborted", "Connection refused", "Not connected", "Already connected", "Connection closed", "Initialization error (interapplication manager)", "Bad occurrence", "Wait on unbound occurrence handler", "Occurrence queue overflow", "Datalog type conflict", "Unused", "Unrecognized type (interapplication manager)", "Memory corrupt", "Failed to make temporary DLL", "Old CIN version", "Drag socket not found", "Failed to load drop-object", "Failed to register OLE object", "Failed to release OLE object", "Format specifier type mismatch", "Unknown format specifier", "Too few format specifiers", "Too many format specifiers", "Scan failed", "Newer CIN version", "Error converting to variant", "Runtime menu error", "Password tampered", "Variant attribute not found", "Incompatible variant data type", "Event data is not available", "Event Store is not present", "Occurrence is not found", "Event Queue is not created", "Event info is not available", "Refnum passed is NULL", "Error retrieving Class GUID", "Error retrieving CoClass GUID", "Error retrieving TypeLib GUID.", "Bad built application magic bytes.", "Specific driver is different from the specific driver associated with the Logical Name.", "There is no session opened to the class driver.", "Max Error", "MAX - Error with config objects", "MAX - Error loading configuration", "MAX - Group not supported"]
        # "Current State"
        # "Do not delete, rename, or modify this frame.\n(this is used to capture unhandled states and typos)"
        # "Handle mistyped state name (developer tool)"
        n157 = Format Into String(format string="Software Exception: Unhandled State \"%s\"." ("message"), error in=w269, w264) -> (resulting string=w272:string, error out=w271:errorcluster)  [unwired: 1 in]
        n158 = call <vilib>:"Error Cluster From Error Code.vi"("show call chain? (False)"=TRUE, "error in (no error)"=w271, "error message (\"\")"=w272, "error code (0)"=w273) -> ("error out"=w270:errorcluster)  [unwired: 5 in]
        n159 = call <vilib>:"Add State(s) to Queue__jki_lib_state_machine.vi"("State(s) in (\"\")"=w268) -> ("States Out"=w267:string)  [unwired: 14 in]
      }
      frame "Initialize Core Data" {
        # "Do not delete, rename, or modify this frame.\n(this is used to determine panel behavior on exit)"
        # "originally closed?"
        # "exe?"
        # "If panel starts closed or is an EXE, then close it when we exit"
        n160 = property class="VI"() -> ("Front Panel.Open"=w282:bool)  [unwired: 2 in, 2 out]
        n161 = property class="App"() -> ("App.Kind"=w281:T5)  [unwired: 2 in, 2 out]
        n162 = control-ref of="Current VI Reference"() -> (w275:refnum<vi>)
        n163 = Not(x=w282) -> (.not. x?=w279:bool)
        n164 = Equal?(x=w281, y=T5."Run Time System" ("Application:Kind")) -> (x = y?=w278:bool)
        n165 = Or(x=w279, y=w278) -> (x .or. y?=w276:bool)
        n166 = Bundle By Name(cluster=w277, "Core.Current VI Reference"=w275, "Core.Close Panel on Exit?"=w276) -> (w284:T10)
        n167 = call <vilib>:"Add State(s) to Queue__jki_lib_state_machine.vi"("State(s) in (\"\")"=w286) -> ("States Out"=w285:string)  [unwired: 14 in]
      }
      frame "Error Handler" {
        # "Unhandled Error -- Display it"
        # "Handle any errors here.\nYou can also output any states to clean-up after errors occur"
        # "Clear error"
        n168 = Wait (ms)(milliseconds to wait=u32 1500) -> ()  [unwired: 1 out]
        n169 = call <vilib>:"Add State(s) to Queue__jki_lib_state_machine.vi"("State(s) in Front (\"\")"="/* Post Error States", "State(s) in (\"\")"=w293) -> ("States Out"=w292:string)  [unwired: 13 in]
        "error out 5" <- w287
      }
      frame "Exit" {
        # "Do not put any code in this frame.\n(No errors that occur here will be handled.)"
        n170 = call <vilib>:"Add State(s) to Queue__jki_lib_state_machine.vi"("State(s) in (\"\")"=w298) -> ("States Out"=w297:string)  [unwired: 14 in]
      }
      frame "---------- Data ----------" {
        # "Do not put any code in this frame.\n(It is a separator no-op. You can make a copy of this frame to create a new Data frame)"
        n171 = call <vilib>:"Add State(s) to Queue__jki_lib_state_machine.vi"("State(s) in (\"\")"=w302) -> ("States Out"=w301:string)  [unwired: 14 in]
      }
      frame "Data: Initialize" {
        # "Initialize the shift-register data, here.\n(data names are defined by what you wire into the bundle function)"
        n172 = call "Data Cluster Plotter.vi"() -> ("output cluster"=w303:T10)
        n173 = call <vilib>:"Add State(s) to Queue__jki_lib_state_machine.vi"("State(s) in (\"\")"=w306) -> ("States Out"=w305:string)  [unwired: 14 in]
      }
      frame "Data: Cleanup" {
        # "Cleanup any data and references, here.\n(this is called automatically, by the Macro: Exit)"
        n174 = Unbundle By Name(w307) -> ("Core.Current VI Reference"=w310:refnum<vi>)
        n175 = Close Reference(reference=w310, error in (no error)=w309) -> (error out=w308:errorcluster)
        n176 = call <vilib>:"Add State(s) to Queue__jki_lib_state_machine.vi"("State(s) in (\"\")"=w312) -> ("States Out"=w311:string)  [unwired: 14 in]
      }
      frame "---------- UI ----------" {
        # "Do not put any code in this frame.\n(It is a separator no-op. You can make a copy of this frame to create a new UI frame)"
        n177 = call <vilib>:"Add State(s) to Queue__jki_lib_state_machine.vi"("State(s) in (\"\")"=w316) -> ("States Out"=w315:string)  [unwired: 14 in]
      }
      frame "UI: Initialize" {
        # "Initialize the User Interface, here.\n(this is called automatically, by the Macro: Init)"
        n178 = call <vilib>:"Add State(s) to Queue__jki_lib_state_machine.vi"("State(s) in (\"\")"=w320) -> ("States Out"=w319:string)  [unwired: 14 in]
      }
      frame "UI: Cursor Set" {
        # "Argument"
        # "Set and Unset Cursor Busy.\n(Usage: \"UI: Cursor Set >> Busy|Idle\")"
        n179 = case shown="\"Idle\", Default" w321 {
          tunnel: w323 -> [w328 w330]
          tunnel: [w327 w329] -> w322
          frame "Idle", Default {
            n180 = call <vilib>:"Unset Busy.vi"("error in (no error)"=w328) -> ("error out"=w327:errorcluster)  [unwired: 10 in]
          }
          frame "Busy" {
            n181 = call <vilib>:"Set Busy.vi"("error in (no error)"=w330) -> ("error out"=w329:errorcluster)  [unwired: 9 in, 1 out]
          }
        }
        n182 = call <vilib>:"Add State(s) to Queue__jki_lib_state_machine.vi"("State(s) in (\"\")"=w326) -> ("States Out"=w325:string)  [unwired: 14 in]
      }
      frame "UI: Front Panel State" {
        # "Argument"
        # "Set Front Panel Open or Closed\n(Usage: \"UI: Front Panel State >> Open|Close\")"
        n183 = Unbundle By Name(w333) -> ("Core.Current VI Reference"=w332:refnum<vi>)
        n184 = case shown="\"Open\", Default" w331 {
          tunnel: w335 -> [w341 w354]
          tunnel: [w343 w355] -> w334
          tunnel: w332 -> [w342 w352]
          frame "Open", Default {
            n185 = property class="VI"(reference=w342, error in=w341) -> (reference out=w339:refnum<vi>, error out=w340:errorcluster, "Front Panel.Open"=w338:bool)
            n186 = case shown="True" w338 {
              tunnel: [w346 w349] -> w343
              tunnel: w340 -> [w345 w349]
              tunnel: w339 -> [w344 _]
              frame False {
                n187 = invoke class="VI" method="FP.Open"(reference=w344, error in=w345, "Activate"=TRUE, "State"=T6."Standard") -> (error out=w346:errorcluster)  [unwired: 1 in, 4 out]
              }
              frame True {
              }
            }
          }
          frame "Close" {
            n188 = property class="VI"(reference=w352, error in=w354) -> (reference out=w351:refnum<vi>, error out=w353:errorcluster, "Front Panel.Open"=w350:bool)
            n189 = case shown="True" w350 {
              tunnel: [w356 w359] -> w355
              tunnel: w353 -> [w356 w358]
              tunnel: w351 -> [_ w357]
              frame False {
              }
              frame True {
                n190 = invoke class="VI" method="FP.Close"(reference=w357, error in=w358) -> (error out=w359:errorcluster)  [unwired: 1 in, 2 out]
              }
            }
          }
        }
        n191 = call <vilib>:"Add State(s) to Queue__jki_lib_state_machine.vi"("State(s) in (\"\")"=w337) -> ("States Out"=w336:string)  [unwired: 14 in]
      }
      frame "---------- Macro ----------" {
        # "Do not put any code in this frame.\n(It is a separator no-op. You can make a copy of this frame to create a new Macro frame)"
        n192 = call <vilib>:"Add State(s) to Queue__jki_lib_state_machine.vi"("State(s) in (\"\")"=w363) -> ("States Out"=w362:string)  [unwired: 14 in]
      }
      frame "Macro: Initialize" {
        w365 = "Data: Initialize\nInitialize Core Data\nUI: Initialize\nUI: Front Panel State >> Open\nMain: Macro"  # Data: Initialize Initialize Core Data UI: Initialize UI: Front Panel State >> Open Main: Macro
        # "Initialization Macro\n(This is called once, when the VI starts)"
        n193 = call <vilib>:"Add State(s) to Queue__jki_lib_state_machine.vi"("State(s) in Front (\"\")"=w365, "State(s) in (\"\")"=w368) -> ("States Out"=w367:string)  [unwired: 13 in]
      }
      frame "Macro: Exit" {
        # "Exit Macro\n(This is called once, when the VI exits)"
        n194 = Unbundle By Name(w376) -> ("Core.Close Panel on Exit?"=w375:bool)
        n195 = Select(t="UI: Front Panel State >> Close", s=w375, f="") -> (s? t:f=w372:string)
        n196 = call <vilib>:"Add State(s) to Queue__jki_lib_state_machine.vi"("State(s) in (\"\")"=w372, "State(s) at Back (\"\")"="Data: Cleanup\nExit") -> ("States Out"=w370:string)  [unwired: 13 in]
        n197 = call <vilib>:"Add State(s) to Queue__jki_lib_state_machine.vi"("State(s) in Front (\"\")"=w370, "State(s) in (\"\")"=w378) -> ("States Out"=w377:string)  [unwired: 13 in]
      }
      frame "---------- Main ----------" {
        # "Template Separator\n(You can make a copy of, or modify, this frame)"
        n198 = call <vilib>:"Add State(s) to Queue__jki_lib_state_machine.vi"("State(s) in (\"\")"=w382) -> ("States Out"=w381:string)  [unwired: 14 in]
      }
      frame "Main: Macro" {
        # "Sets the list of states to execute on vi startup in the first string and  the list of states to execute on each loop\nin the second string"
        n199 = local write "Tab Control"(0) -> ()
        n200 = call <vilib>:"Add State(s) to Queue__jki_lib_state_machine.vi"("State(s) in Front (\"\")"="Main: Read Expt Configs\nMain: Get Expt name\nGet plotter details\nMain: Read Expt Config\nGet List of Axis Names\nGet Default Y Axis\nMain: Set Panel Postion\nMain: Get Device Configs", "State(s) in (\"\")"=w388) -> ("States Out"=w387:string)  [unwired: 13 in]
      }
      frame "Main: Read Expt Configs" {
        # "Gets experimental configuration filenames. These files contain information specific to an experiment. Eg TREX expt\nfile would have all the devices that need to startup and their default variable values."
        n201 = call "preset SQL Queries.vi"("error in (no error)"=w390, "Preset Query"=Preset_Query_Enum."Get Expt names") -> ("error out"=w389:errorcluster, "1st column 1st data"=w391:string[])  [unwired: 7 in, 1 out]
        n202 = call "array to strings and values for ring.vi"("list of variables"=w391) -> ("Array"=w395:cluster{"String":string, i32}[])
        n203 = property on="Experiment" class="Ring (strict)"("StringsAndValues[]"=w395) -> ()  [unwired: 2 in, 2 out]
        n204 = Bundle By Name(cluster=w394, "Expt Config Files"=w391) -> (w393:T10)
        n205 = call <vilib>:"Add State(s) to Queue__jki_lib_state_machine.vi"("State(s) in (\"\")"=w397) -> ("States Out"=w396:string)  [unwired: 14 in]
      }
      frame "Main: Get Expt name" {
        # "cmd is ...plotter.exe>>plotterid#"
        # "Increments scan #, resets shot number and sends list of states to execute at the start of a scan. Only does this\nif variable for scan is numeric."
        n206 = disable-structure shown="default" {
          disable-tunnel: ["expt_Plotteridfor vi mode" w425] -> w398
          disable-tunnel: [_ w420] -> w402
          disable-tunnel: [_ w419] -> w400
          frame condition #0 (active) {
          }
          frame condition #1 {
            n207 = control-ref of="This Application"() -> (w426:refnum<vi>)
            n208 = property class="App"(reference=w426) -> ("App.Args"=w424:string[])  [unwired: 1 in, 2 out]
            "appargs" <- w424
            n209 = Index Array(array=w424, index #1=2 ("index"), index #2=3 ("index"), index #3=4 ("index")) -> (element #1=w425:string, element #2=w420:string, element #3=w419:string)
          }
        }
        "Actual expt_plotter.id" <- w398
        n210 = Unbundle By Name(w415) -> ("Expt Config Files"=w413:string[])
        n211 = property on="Experiment" class="Ring (strict)"() -> ("Strings []"=w407:string[])  [unwired: 2 in, 2 out]
        n212 = call "preset SQL Queries.vi"("error in (no error)"=w404, "Device/Devicetype name\n/Plotter.id/ScanName#"=w398, "Preset Query"=Preset_Query_Enum."Get expt for plotter") -> ("error out"=w403:errorcluster, "data"=w410:string[][])  [unwired: 6 in, 1 out]
        n213 = Index Array(array=w410, index (row)=1) -> (element=w412:string[])  [unwired: 1 in]
        n214 = Decimal String To Number(string=w402) -> (number=w401:i32)  [unwired: 2 in, 1 out]
        n215 = Decimal String To Number(string=w400) -> (number=w399:i32)  [unwired: 2 in, 1 out]
        n216 = Index Array(array=w412) -> (element #1=w405:string, element #2=w408:string)  [unwired: 2 in]
        "expt" <- w405
        "plotter#" <- w408
        n217 = Search 1D Array(1D array=w407, element=w405) -> (index of element=w406:i32)  [unwired: 1 in]
        "Experiment" <- w406
        n218 = Index Array(array=w413, index=w406) -> ()  [unwired: 1 out]
        n219 = Bundle By Name(cluster=w415, "Experiment name"=w405, "plotter#"=w408, "Plotter setup cluster.screenx"=w401, "Plotter setup cluster.screeny"=w399) -> (w414:T10)
        n220 = call <vilib>:"Add State(s) to Queue__jki_lib_state_machine.vi"("State(s) in (\"\")"=w417) -> ("States Out"=w416:string)  [unwired: 14 in]
      }
      frame "Get plotter details" {
        # "Template Separator\n(You can make a copy of, or modify, this frame)"
        n221 = Unbundle By Name(w432) -> ("plotter#"=w442:string)
        n222 = call "preset SQL Queries.vi"("error in (no error)"=w429, "Device/Devicetype name\n/Plotter.id/ScanName#"=w442, "Preset Query"=Preset_Query_Enum."Get plotter details") -> ("error out"=w428:errorcluster, "data"=w441:string[][])  [unwired: 6 in, 1 out]
        "plotter details" <- w441
        n223 = Index Array(array=w441, index (row)=1) -> (element=w439:string[])  [unwired: 1 in]
        n224 = Index Array(array=w439) -> (element #2=w438:string, element #3=w436:string, element #4=w434:string, element #5=w433:string, element #6=w427:string)  [unwired: 6 in, 1 out]
        n225 = Decimal String To Number(string=w438) -> (number=w437:i32)  [unwired: 2 in, 1 out]
        n226 = Decimal String To Number(string=w436) -> (number=w435:i32)  [unwired: 2 in, 1 out]
        n227 = Bundle By Name(cluster=T8 {"screenx"=25, "screeny"=75, "variable1"="", "variable2"="", "name"=""} ("Plotter setup cluster"), "screenx"=w437, "screeny"=w435, "variable1"=w434, "variable2"=w433, "name"=w427) -> (w430:T8)
        n228 = Bundle By Name(cluster=w432, "Plotter setup cluster"=w430) -> (w431:T10)
        n229 = call <vilib>:"Add State(s) to Queue__jki_lib_state_machine.vi"("State(s) in (\"\")"=w446) -> ("States Out"=w445:string)  [unwired: 14 in]
      }
      frame "Main: Read Expt Config" {
        # "todo. get rid of the copy of parameters"
        # "Reads the configuration for a particular experiment. eg TREX default would save spectrum mode image and\nget back centroid etc."
        n230 = Unbundle By Name(w473) -> ("Experiment name"=w455:string)
        n231 = call "preset SQL Queries.vi"("error in (no error)"=w454, "Expt name / MCIP/ Variable/Preset Name"=w455, "Preset Query"=Preset_Query_Enum."Get experiment basic properties") -> ("error out"=w453:errorcluster, "1st column 1st data"=w451:string[], "data"=w450:string[][])  [unwired: 6 in]
        n232 = Index Array(array=w451) -> (element=w457:string)  [unwired: 1 in]
        n233 = Index Array(array=w450, index (row)=1, index (col)=2 ("disabled index (col)")) -> (element=w447:string)
        n234 = call "preset SQL Queries.vi"("error in (no error)"=w453, "Expt name / MCIP/ Variable/Preset Name"=w455, "Preset Query"=Preset_Query_Enum."Get expt devices with data to get") -> ("error out"=w471:errorcluster, "data"=w468:string[][])  [unwired: 6 in, 1 out]
        n235 = Decimal String To Number(string=w447) -> (number=w452:i32)  [unwired: 2 in, 1 out]
        n236 = Delete From Array(array=w468, index (row)=0) -> (array with subset deleted=w470:string[][])  [unwired: 2 in, 1 out]
        n237 = Index Array(array=w470, index (col)=0 ("disabled index (col)")) -> (element=w463:string[])  [unwired: 1 in]
        "devices to get data from" <- w463
        n238 = call "preset SQL Queries.vi"("error in (no error)"=w471, "Expt name / MCIP/ Variable/Preset Name"=w455, "Preset Query"=Preset_Query_Enum."Get expt devices and variables (with data to get)") -> ("error out"=w464:errorcluster, "data"=w462:string[][])  [unwired: 6 in, 1 out]
        "parameters to get" <- w462
        n239 = Bundle By Name(cluster=w473, "expt config file array"=w462, "ScanData to receive"=w462, "Device Names for scan data"=w463) -> (w472:T10)
        n240 = call "Plotter FGV Cluster.vi"("Function"=enum16{"Read", "Write", "Clear"}."Read") -> ("Cluster out"=w458:T4)  [unwired: 9 in, 1 out]
        n241 = Bundle By Name(cluster=w458, "Multicast Address"=w457, "Mcast Port"=w452) -> (w456:T4)
        n242 = call <vilib>:"Add State(s) to Queue__jki_lib_state_machine.vi"("State(s) in (\"\")"=w475) -> ("States Out"=w474:string)  [unwired: 14 in]
        n243 = call "Plotter FGV Cluster.vi"("Function"=enum16{"Read", "Write", "Clear"}."Write", "Cluster in"=w456) -> ()  [unwired: 8 in, 2 out]
      }
      frame "Get List of Axis Names" {
        # "Increments scan #, resets shot number and sends list of states to execute at the start of a scan. Only does this\nif variable for scan is numeric."
        n244 = Unbundle By Name(w481) -> ("ScanData to receive"=w479:string[][])
        n245 = Delete From Array(array=w479, index (row)=0) -> (array with subset deleted=w477:string[][])  [unwired: 2 in, 1 out]
        n246 = Index Array(array=w477, index (col) #1=0 ("disabled index (col)"), index (col) #2=1 ("index (col)")) -> (element #1=w483:string[], element #2=w482:string[])  [unwired: 2 in]
        n247 = for {
          tunnel: w483 -> [w491] mode=indexing
          tunnel: w482 -> [w490] mode=indexing
          tunnel: [w489] -> w476 mode=indexing
          n248 = Concatenate Strings(w491, " " ("string"), w490) -> (w489:string)
        }
        "Axis Name List" <- w476
        n249 = Bundle By Name(cluster=w481, "Data titles from config array"=w476) -> (w480:T10)
        n250 = property on="Y Axis 2" class="Ring (strict)"("Strings []"=w476) -> ()  [unwired: 2 in, 2 out]
        n251 = property on="Y Axis" class="Ring (strict)"("Strings []"=w476) -> ()  [unwired: 2 in, 2 out]
        n252 = property on="X Axis" class="Ring (strict)"("Strings []"=w476) -> ()  [unwired: 2 in, 2 out]
        n253 = call <vilib>:"Add State(s) to Queue__jki_lib_state_machine.vi"("State(s) in (\"\")"=w488) -> ("States Out"=w487:string)  [unwired: 14 in]
      }
      frame "Get Default Y Axis" {
        # "Increments scan #, resets shot number and sends list of states to execute at the start of a scan. Only does this\nif variable for scan is numeric."
        n254 = Unbundle By Name(w501) -> ("Plotter setup cluster.variable1"=w496:string, "Plotter setup cluster.variable2"=w495:string)
        "Y Axis Default name" <- w496
        n255 = stacked-sequence {
          tunnel: w496 -> [w508 w512]
          tunnel: w495 -> [w507 w511]
          tunnel: 0 ("Active Y Scale") -> [w506 w510]
          tunnel: 1 ("Active Y Scale") -> [w505 w509]
          frame #0 {
            n256 = property on="xy graph" class="XYGraph (strict)"("ActYScl"=w506, "YScale.NameLbl.Text"=w508, "ActYScl"=w505, "YScale.NameLbl.Text"=w507) -> ()  [unwired: 2 in, 2 out]
          }
          frame #1 {
            n257 = property on="xy graph bin" class="XYGraph (strict)"("ActYScl"=w510, "YScale.NameLbl.Text"=w512, "ActYScl"=w509, "YScale.NameLbl.Text"=w511) -> ()  [unwired: 2 in, 2 out]
          }
        }
        n258 = property on="Y Axis" class="Ring (strict)"() -> ("Strings []"=w500:string[])  [unwired: 2 in, 2 out]
        n259 = property on="Y Axis 2" class="Ring (strict)"() -> ("Strings []"=w498:string[])  [unwired: 2 in, 2 out]
        n260 = Search 1D Array(1D array=w498, element=w495) -> (index of element=w497:i32)  [unwired: 1 in]
        n261 = Search 1D Array(1D array=w500, element=w496) -> (index of element=w499:i32)  [unwired: 1 in]
        n262 = local write "Y Axis"(w499) -> ()
        n263 = local write "Y Axis 2"(w497) -> ()
        n264 = call <vilib>:"Add State(s) to Queue__jki_lib_state_machine.vi"("State(s) in (\"\")"=w504) -> ("States Out"=w503:string)  [unwired: 14 in]
      }
      frame "open tcp connections" {
        # "Your code here.\n(You can make a copy of, or modify, this frame)"
        n265 = disable-structure shown="Enabled" {
          disable-tunnel: w517 -> [w547 w568]
          disable-tunnel: w516 -> [w527 _]
          disable-tunnel: [w526 _] -> w515
          disable-tunnel: [w522 w565] -> w514
          disable-tunnel: [w526 _] -> w513
          frame Enabled {
            w521 = "Shot #" ("Active Variable")
            w529 = 1000 ("timeout ms (60000)")
            n266 = local read "x axis name"() -> (w524:string)
            n267 = Unbundle By Name(w547) -> ("Plotter setup cluster.variable1"=w546:string, "Plotter setup cluster.variable2"=w541:string)
            n268 = Equal?(x=w524, y=w521) -> (x = y?=w525:bool)
            "shotoverride" <- w525
            n269 = Search/Split String(string=w546, search string/char (-)=" ") -> (substring before match=w544:string, match + rest of string=w543:string)  [unwired: 1 in, 1 out]
            n270 = call "subscribe command.vi"("variable"=w541) -> ("IP"=w539:string, "port"=w537:string, "subscribe command"=w531:string)
            n271 = String Subset(string=w543, offset (0)=1) -> (substring=w533:string)  [unwired: 1 in]
            n272 = call "get device ip and port.vi"("variable1"=w544) -> ("port"=w538:string, "IP"=w540:string)  [unwired: 1 out]
            n273 = Build Array(w540, w539) -> (w536:string[])
            "ipjjj" <- w536
            n274 = Build Array(w538, w537) -> (w535:string[])
            "portrsvvv" <- w535
            n275 = Concatenate Strings("Wait>>" ("search string/char (-)"), w533) -> (w532:string)
            n276 = call "TCP multiple open.vi"("timeout ms (60000)"=w529, "Ports"=w535, "error in 1 (no error)"=w527, "IP Addresses"=w536) -> ("error out"=w528:errorcluster, "Array"=w523:refnum<k5>[])  [unwired: 1 out]
            n277 = case shown="True" w525 {
              tunnel: w524 -> [w548 _]
              tunnel: [w549 w564] -> w522
              tunnel: w523 -> [w551 w564]
              tunnel: w521 -> [_ w563]
              frame False {
                w552 = 1000 ("timeout ms (60000)")
                n278 = call "subscribe command.vi"("variable"=w548) -> ("IP"=w559:string, "port"=w560:string, "subscribe command"=w553:string)
                "subscribe command" <- w553
                n279 = Decimal String To Number(string=w560) -> (number=w562:i32)  [unwired: 2 in, 1 out]
                n280 = property on="xy graph" class="XYGraph (strict)"("XScale.NameLbl.Text"=w548) -> ()  [unwired: 2 in, 2 out]
                n281 = To Unsigned Word Integer(number=w562) -> (unsigned 16bit integer=w561:u16)
                n282 = property on="xy graph bin" class="XYGraph (strict)"("XScale.NameLbl.Text"=w548) -> ()  [unwired: 2 in, 2 out]
                n283 = TCP Open Connection(address=w559, remote port or service name=w561, timeout ms (60000)=w552) -> (connection ID=w554:refnum<k5>)  [unwired: 2 in, 1 out]
                n284 = String Length(string=w553) -> (length=w557:i32)
                n285 = Type Cast(type=w553, x=w557) -> (*(type *) &x=w558:string)
                n286 = TCP Write(connection ID=w554, data in=w558) -> (connection ID out=w555:refnum<k5>, error out=w556:errorcluster)  [unwired: 2 in, 1 out]
                n287 = TCP Write(connection ID=w555, data in=w553, error in (no error)=w556, 9:w552) -> (connection ID out=w550:refnum<k5>)  [unwired: 2 out]
                n288 = Build Array (concatenate)(w551, w550) -> (w549:refnum<k5>[])
              }
              frame True {
                n289 = property on="xy graph" class="XYGraph (strict)"("XScale.NameLbl.Text"=w563) -> ()  [unwired: 2 in, 2 out]
                n290 = local write "x axis name"(w563) -> ()
                n291 = property on="xy graph bin" class="XYGraph (strict)"("XScale.NameLbl.Text"=w563) -> ()  [unwired: 2 in, 2 out]
              }
            }
            n292 = Build Array(w532, w531) -> (w530:string[])
            "appended array" <- w530
            n293 = call "tcp multiple write.vi"("Connection ID array"=w523, "error in 1 (no error)"=w528, "messages to send"=w530, "timeout ms (25000)"=w529) -> ("error out"=w526:errorcluster)
          }
          frame Disabled {
            n294 = Unbundle By Name(w568) -> ("All Devices Core Info"=w567:string[][], "Device Names for scan data"=w566:string[], "ScanData to receive"=w576:string[][])
            "ScanData to receive" <- w576
            n295 = call "get info from core device data.vi"("devices to get data from"=w566, "All Devices Core Info"=w567) -> ("Ports"=w575:string[], "IP Addresses"=w569:string[])  [unwired: 2 in]
            "udp ports to listen to" <- w575
            "IPs" <- w569
            n296 = call "scan data to receive to subscribe commands.vi"("ScanData to receive"=w576) -> ("Subscribe commands"=w574:string[])  [unwired: 8 in, 2 out]
            n297 = call "TCP multiple open.vi"("timeout ms (60000)"="TCP Open timeout ms", "Ports"=w575, "IP Addresses"=w569) -> ("error out"=w571:errorcluster, "Array"=w565:refnum<k5>[])  [unwired: 1 in]
            n298 = call "tcp multiple write.vi"("Connection ID array"=w565, "error in 1 (no error)"=w571, "messages to send"=w574, "timeout ms (25000)"=300) -> ("error out"=→"TCP scan error out":errorcluster)
          }
        }
        n299 = case shown="Error" w513 {
          tunnel: w514 -> [w520 _]
          frame No Error {
            "TCP Ports" <- w520
          }
          frame Error {
          }
        }
        n300 = call <vilib>:"Add State(s) to Queue__jki_lib_state_machine.vi"("State(s) in (\"\")"=w519) -> ("States Out"=w518:string)  [unwired: 14 in]
      }
      frame "Main: Set Panel Postion" {
        # "Reads the configuration for a particular experiment. eg TREX default would save spectrum mode image and\nget back centroid etc."
        n301 = Unbundle By Name(w586) -> ("Plotter setup cluster.screenx"=w582:i16, "Plotter setup cluster.screeny"=w581:i16)
        n302 = property on="Tab Control" class="TabCtl (strict)"() -> ("PaneWidth"=w590:u32, "PaneHeight"=w589:u32)  [unwired: 2 in, 2 out]
        n303 = Add(x=w589, y=u32 25) -> (x+y=w579:u32)
        n304 = Add(x=u32 15, y=w590) -> (x+y=w580:u32)
        n305 = call <vilib>:"Add State(s) to Queue__jki_lib_state_machine.vi"("State(s) in (\"\")"=w592) -> ("States Out"=w591:string)  [unwired: 14 in]
        n306 = Bundle By Name(cluster="Cluster", "Left"=w582, "Top"=w581, "Width"=w580, "Height"=w579) -> (w584:T1)
        n307 = control-ref of="This VI"() -> (w583:refnum<vi>)
        n308 = call "set panel position MC only.vi"("error out 2"=w578, "Cluster"=w584, "This VI"=w583) -> ("error out"=w577:errorcluster)
      }
      frame "Main: Get Device Configs" {
        # "Reads the configuration for a particular experiment. eg TREX default would save spectrum mode image and\nget back centroid etc."
        n309 = call "preset SQL Queries.vi"("error in (no error)"=w594, "Preset Query"=Preset_Query_Enum."Get all devices basic properties") -> ("error out"=w593:errorcluster, "data"=w595:string[][])  [unwired: 7 in, 1 out]
        "All Devices Core Info" <- w595
        n310 = Bundle By Name(cluster=w597, "All Devices Core Info"=w595) -> (w598:T10)
        n311 = call <vilib>:"Add State(s) to Queue__jki_lib_state_machine.vi"("State(s) in (\"\")"=w600) -> ("States Out"=w599:string)  [unwired: 14 in]
      }
      frame "Plot" {
        # "Your code here.\n(You can make a copy of, or modify, this frame)"
        n312 = Unbundle By Name(w623) -> ("TDMS file path"=w621:path)
        "TDMS file path" <- w621
        n313 = call "Plotter FGV Cluster.vi"("error in"=w605, "Function"=enum16{"Read", "Write", "Clear"}."Read") -> ("error out"=w612:errorcluster, "Cluster out"=w614:T4)  [unwired: 8 in]
        n314 = Bundle By Name(cluster=w614, "Plotter Busy"=TRUE) -> (w611:T4)
        n315 = Select(t="file path", s="FilePath", f=w621) -> (s? t:f=w620:path)
        "Path used" <- w620
        n316 = call "Plotter FGV Cluster.vi"("error in"=w612, "Function"=enum16{"Read", "Write", "Clear"}."Write", "Cluster in"=w611) -> ("error out"=w616:errorcluster, "Cluster out"=w608:T4)  [unwired: 7 in]
        n317 = Bundle By Name(cluster=w608, "Plotter Busy"=FALSE) -> (w607:T4)
        n318 = call <vilib>:"Check if File or Folder Exists.vi"("error in (no error)"=w616, "path"=w620) -> ("error out"=w617:errorcluster, "file or folder exists?"=w619:bool, "dup path"=w618:path)  [unwired: 7 in]
        n319 = case shown="True" w619 {
          tunnel: w618 -> [_ w636]
          tunnel: w623 -> [_ w639]
          tunnel: w617 -> [w626 w628]
          tunnel: w603 -> [_ w638]
          tunnel: "FilePath" -> [_ w637]
          tunnel: [w626 w627] -> w601
          frame False {
          }
          frame True {
            # "todo. use multiple bin"
            n320 = local read "shot# 2"() -> (w630:i32)
            n321 = local read "y2"() -> (w634:dbl[])
            n322 = local read "y1"() -> (w632:dbl[])
            n323 = Array Subset(array=w632, index=1, length=w630) -> (w629:dbl[])
            n324 = Array Subset(array=w634, index=1, length=w630) -> (w633:dbl[])
            n325 = stacked-sequence {
              seq-local: [w640 _ _ _ _] -> [_ _ _ w667 w709]
              seq-local: [_ _ _ w666 _] -> [_ _ _ _ _]
              tunnel: w636 -> [w647 _ _ w672 w715]
              tunnel: w639 -> [_ w661 _ _ w714]
              tunnel: w638 -> [_ _ _ _ w716]
              tunnel: w637 -> [_ _ _ w670 _]
              tunnel: w633 -> [w642 _ _ w669 _]
              tunnel: w629 -> [_ _ _ w668 _]
              tunnel: w628 -> [w641 _ _ _ _]
              tunnel: [_ _ _ _ w708] -> w627
              frame #0 {
                n326 = Array Size(array=w642) -> (size(s)=w646:i32)
                n327 = In Range and Coerce(upper limit=4 ("y"), x=w646, lower limit=2) -> (In Range?=w644:bool)  [unwired: 1 out]
                n328 = case shown="True" w644 {
                  tunnel: w647 -> [_ w651]
                  tunnel: w641 -> [w648 w650]
                  tunnel: [w648 w649] -> w640
                  frame False {
                  }
                  frame True {
                    n329 = call "Read TDMS - LOASIS scan data.vi"("error in (no error)"=w650, "file path"=w651) -> ("error out"=w649:errorcluster, "device data Spreadsheet format"=w654:string[][])  [unwired: 8 in]
                    n330 = Index Array(array=w654, index (row)=0) -> (element=w652:string[])  [unwired: 1 in]
                    n331 = property on="Y Axis 2" class="Ring (strict)"("Strings []"=w652) -> ()  [unwired: 2 in, 2 out]
                    n332 = property on="X Axis" class="Ring (strict)"("Strings []"=w652) -> ()  [unwired: 2 in, 2 out]
                    n333 = property on="Y Axis" class="Ring (strict)"("Strings []"=w652) -> ()  [unwired: 2 in, 2 out]
                  }
                }
              }
              frame #1 {
                n334 = Unbundle By Name(w661) -> ("Plotter setup cluster.variable1"=w659:string, "Plotter setup cluster.variable2"=w656:string)
                n335 = property on="Y Axis 2" class="Ring (strict)"() -> ("Strings []"=w657:string[])  [unwired: 2 in, 2 out]
                n336 = property on="Y Axis" class="Ring (strict)"() -> ("Strings []"=w660:string[])  [unwired: 2 in, 2 out]
                n337 = Search 1D Array(1D array=w657, element=w656) -> (index of element=w655:i32)  [unwired: 1 in]
                n338 = Search 1D Array(1D array=w660, element=w659) -> (index of element=w658:i32)  [unwired: 1 in]
                n339 = local write "Y Axis 2"(w655) -> ()
                n340 = local write "Y Axis"(w658) -> ()
              }
              frame #2 {
                n341 = local read "FilePath"() -> (w662:bool)
                n342 = case shown="False" w662 {
                  frame False {
                    n343 = local read "x axis name"() -> (w664:string)
                    n344 = property on="X Axis" class="Ring (strict)"() -> ("Strings []"=w665:string[])  [unwired: 2 in, 2 out]
                    n345 = Search 1D Array(1D array=w665, element=w664) -> (index of element=w663:i32)  [unwired: 1 in]
                    n346 = local write "X Axis"(w663) -> ()
                  }
                  frame True {
                  }
                }
              }
              frame #3 {
                n347 = case shown="False" w670 {
                  tunnel: w672 -> [_ w699]
                  tunnel: [w689 w707] -> w671
                  tunnel: w669 -> [w678 _]
                  tunnel: w668 -> [w675 _]
                  tunnel: w667 -> [w673 w698]
                  tunnel: [w673 w697] -> w666
                  frame False {
                    w674 = 1000 ("max array size")
                    n348 = local read "shotoverride"() -> (w687:bool)
                    n349 = local read "shot# 2"() -> (w684:i32)
                    n350 = local read "shot#"() -> (w685:i32)
                    n351 = Greater?(x=w685, y=w684) -> (0:w686:bool)
                    n352 = Select(t=w685, s=w686, f=w684) -> (s? t:f=w683:i32)
                    n353 = case shown="False" w687 {
                      tunnel: [w690 w695] -> w688
                      tunnel: w683 -> [_ w694]
                      frame False {
                        n354 = local read "x"() -> (w693:dbl[])
                        n355 = Delete From Array(array=w693, length=1, index=0) -> (array with subset deleted=w690:dbl[])  [unwired: 1 out]
                      }
                      frame True {
                        n356 = call-poly <vilib>:"Ramp Pattern.vi"("start"=1.0, "end"=w694, "samples"=w694) -> ("Ramp Pattern"=w695:dbl[])  [unwired: 7 in, 1 out]
                      }
                    }
                    n357 = call <vilib>:"Std Deviation and Variance.vi"("X"=w678) -> ("mean"=→"RHS mean":dbl, "standard deviation"=→"RHS sigma":dbl)  [unwired: 1 in, 1 out]
                    n358 = call "decimate array max points.vi"("max array size"=w674, "Array in"=w678) -> ("Decimated Array out"=w677:dbl[])  [unwired: 9 in]
                    n359 = call "decimate array max points.vi"("max array size"=w674, "Array in"=w675) -> ("Decimated Array out"=w676:dbl[])  [unwired: 9 in]
                    n360 = call <vilib>:"Std Deviation and Variance.vi"("X"=w675) -> ("mean"=→"LHS mean":dbl, "standard deviation"=→"LHS sigma":dbl)  [unwired: 1 in, 1 out]
                    n361 = call "xy graph from 1d arrays.vi"("y2"=w677, "y1"=w676, "shot#"=w683, "x"=w688) -> ("xy graph"=w689:cluster{"Ramp Pattern":dbl[], dbl[]}[])
                  }
                  frame True {
                    n362 = control-ref of="xy graph"() -> (w706:refnum<vi>)
                    n363 = control-ref of="Y Axis 2"() -> (w705:refnum<vi>)
                    n364 = call "Read TDMS - LOASIS scan data.vi"("error in (no error)"=w698, "file path"=w699) -> ("error out"=w697:errorcluster, "device data Spreadsheet format"=w700:string[][])  [unwired: 8 in]
                    n365 = control-ref of="Y Axis"() -> (w704:refnum<vi>)
                    n366 = control-ref of="X Axis"() -> (w703:refnum<vi>)
                    n367 = Bundle By Name(cluster=T9 {"Ring Refnum x"=refnum, "Ring Refnum y"=refnum, "Ring Refnum y 2"=refnum, "XY Graph Refnum"=refnum} ("Cluster"), "Ring Refnum x"=w703, "Ring Refnum y"=w704, "Ring Refnum y 2"=w705, "XY Graph Refnum"=w706) -> (w701:T9)
                    n368 = call "Select axes.vi"("Cluster"=w701, "output array"=w700) -> ("XY Graph"=w707:cluster{dbl[], dbl[]}[])  [unwired: 4 in, 2 out]
                  }
                }
                "xy graph" <- w671
              }
              frame #4 {
                n369 = Unbundle By Name(w714) -> ("Plotter setup cluster.variable1"=w712:string, "Plotter setup cluster.variable2"=w713:string, "Plotter setup cluster.name"=w710:string)
                n370 = local read "x axis name"() -> (w711:string)
                n371 = case shown="\"nobin\", Default" w716 {
                  tunnel: w715 -> [_ w732]
                  tunnel: w713 -> [_ w724]
                  tunnel: w712 -> [_ w726]
                  tunnel: w711 -> [_ w723]
                  tunnel: w710 -> [_ w731]
                  tunnel: w709 -> [w717 w719]
                  tunnel: [w717 w718] -> w708
                  frame "nobin", Default {
                  }
                  frame "bin" {
                    n372 = call "Read TDMS - LOASIS scan data.vi"("error in (no error)"=w719, "file path"=w732) -> ("error out"=w733:errorcluster, "device data Spreadsheet format"=w725:string[][])  [unwired: 8 in]
                    "device data Spreadsheet format" <- w725
                    n373 = call "binbyStepIndex02.vi"("y1 col name"=w726, "x col name"=w723, "device data Spreadsheet format"=w725) -> ("XY Graph 2"=w722:cluster{"ind":dbl[], "ini2":dbl[]}[])  [unwired: 6 in, 2 out]
                    n374 = call "binbyStepIndex02.vi"("y1 col name"=w724, "x col name"=w723, "device data Spreadsheet format"=w725) -> ("XY Graph 2"=w721:cluster{"ind":dbl[], "ini2":dbl[]}[])  [unwired: 6 in, 2 out]
                    n375 = Build Array (concatenate)(w722, w721) -> (→"xy graph bin":cluster{"ind":dbl[], "ini2":dbl[]}[])
                    n376 = call "tdms path to plotter png path.vi"("error in"=w733, "plotter name"=w731, "TDMS Path"=w732) -> ("error out"=w718:errorcluster, "binned plotter png save path"=w728:path, "plotter png save path"=w727:path)  [unwired: 6 in]
                    n377 = control-ref of="xy graph bin"() -> (w730:refnum<vi>)
                    n378 = control-ref of="xy graph"() -> (w729:refnum<vi>)
                    n379 = call "plotter save png.vi"("binned plotter png save path"=w728, "plotter png save path"=w727, "XYGraph Refnum in"=w730, "XYGraph in"=w729) -> ()  [unwired: 8 in]
                  }
                }
              }
            }
          }
        }
        n380 = call <vilib>:"Add State(s) to Queue__jki_lib_state_machine.vi"("State(s) in (\"\")"=w625) -> ("States Out"=w624:string)  [unwired: 14 in]
        n381 = call "Plotter FGV Cluster.vi"("error in"=w601, "Function"=enum16{"Read", "Write", "Clear"}."Write", "Cluster in"=w607) -> ("error out"=w604:errorcluster)  [unwired: 7 in, 1 out]
      }
      frame "19" {
        # "Your code here.\n(You can make a copy of, or modify, this frame)"
        n382 = call <vilib>:"Add State(s) to Queue__jki_lib_state_machine.vi"("State(s) in (\"\")"=w737) -> ("States Out"=w736:string)  [unwired: 14 in]
      }
      frame "get panel position" {
        # "Your code here.\n(You can make a copy of, or modify, this frame)"
        n383 = control-ref of="This VI"() -> (w744:refnum<vi>)
        n384 = call "get vi screen position.vi"("error in"=w743, "This VI"=w744) -> ("error out"=w742:errorcluster, "Front Panel Window:Panel Bounds"=w741:T11)  [unwired: 8 in]
        n385 = Unbundle By Name(w741) -> ("Left"=w740:i16, "Top"=w739:i16)
        n386 = Bundle("Left"=w740, "Top"=w739) -> (→"Screen\nPosition":cluster{"Left":i16, "Top":i16})  [unwired: 1 in]
        n387 = call <vilib>:"Add State(s) to Queue__jki_lib_state_machine.vi"("State(s) in (\"\")"=w747) -> ("States Out"=w746:string)  [unwired: 14 in]
      }
    }
    "error out 2" <- w139
  }
  n388 = stacked-sequence "TCP subsrcriptions for scan data" {
    tunnel: w1 -> [_ w752]
    frame #0 {
      n389 = local write "TCP Ports"(refnum<k5>[] [] ("TCP Ports")) -> ()
    }
    frame #1 {
      n390 = control-ref of="shot#"() -> (w755:refnum<vi>)
      n391 = control-ref of="TCP Ports"() -> (w757:refnum<vi>)
      n392 = control-ref of="y1"() -> (w756:refnum<vi>)
      n393 = control-ref of="data out 1"() -> (w750:refnum<vi>)
      n394 = Bundle("TCP Ports"=w757, "y1"=w756, "shot#"=w755, "data out 1"=w750) -> (w754:T12)  [unwired: 1 in]
      n395 = call "Plotter TCP Reader1.vi"("error in"=w752, "timeout ms"="timeout ms", "TCP index"=0, "references"=w754) -> ("error out"=→"error out":errorcluster)  [unwired: 7 in]
    }
  }
  n396 = stacked-sequence "TCP subsrcriptions for scan data" {
    tunnel: w1 -> [_ w763]
    frame #0 {
      n397 = local write "TCP Ports"(refnum<k5>[] [] ("TCP Ports")) -> ()
    }
    frame #1 {
      n398 = control-ref of="TCP Ports"() -> (w767:refnum<vi>)
      n399 = control-ref of="shot# 2"() -> (w765:refnum<vi>)
      n400 = control-ref of="y2"() -> (w766:refnum<vi>)
      n401 = control-ref of="data out 2"() -> (w764:refnum<vi>)
      n402 = Bundle("TCP Ports"=w767, "y2"=w766, "shot# 2"=w765, "data out 2"=w764) -> (w762:T13)  [unwired: 1 in]
      n403 = call "Plotter TCP Reader2.vi"("error in"=w763, "timeout ms"=1000, "TCP index"=1, "references"=w762) -> ("error out"=→"error out 3":errorcluster)  [unwired: 7 in]
    }
  }
  n404 = stacked-sequence "TCP subsrcriptions for scan data" {
    tunnel: w1 -> [_ w771]
    frame #0 {
      n405 = local write "TCP Ports"(refnum<k5>[] [] ("TCP Ports")) -> ()
    }
    frame #1 {
      n406 = control-ref of="TCP Ports"() -> (w775:refnum<vi>)
      n407 = control-ref of="x"() -> (w776:refnum<vi>)
      n408 = control-ref of="data out 3"() -> (w777:refnum<vi>)
      n409 = control-ref of="shot# 3"() -> (w769:refnum<vi>)
      n410 = Bundle("TCP Ports"=w775, "x"=w776, "shot# 3"=w769, "data out 3"=w777) -> (w774:T14)  [unwired: 1 in]
      n411 = call "Plotter TCP Reader3.vi"("error in"=w771, "timeout ms"=1000, "TCP index"=2, "references"=w774) -> ("error out"=→"error out 4":errorcluster)  [unwired: 7 in]
    }
  }
  n412 = disable-structure shown="Disabled" {
    frame Disabled {
      n413 = call "binning for loasis TDMS plotter.vi"() -> ()  [unwired: 11 in, 1 out]
    }
    frame Enabled {
    }
  }
